vi "AO_master_CorrLoop_PD_2D_v3.vi"() -> ()   [LabVIEW 2018]
uses:
  <userlib>/WaveKit.lib/Controls/Wavefront Corrector states - ONE.ctl
  <userlib>/WaveKit.lib/Classes/WavefrontCorrector/WavefrontCorrector.lvclass
  <userlib>/WaveKit.lib/Classes/WavefrontCorrectorSet/WavefrontCorrectorSet.lvclass
  <vilib>/Analysis/1siggen.llb/Ramp Pattern by Samples.vi
  <vilib>/Utility/file.llb/Read From Spreadsheet File (DBL).vi
  <vilib>/Analysis/1siggen.llb/Ramp Pattern by Delta.vi
  <vilib>/Analysis/NI_AALBase.lvlib
panel:
  in  "Tab Control":T1(tab)
  in  "Flip mirror port":tag="Dev1/ao5"
  in  "interaction matrix file":path=path "D:/SystemAlignment/IM_20200816_1sx2_0p5um.aomi"
  in  "Haso configuration file":path=path "C:/Program Files (x86)/Imagine Optic/Configuration Files/HASO3_first_7364.dat"
  in  "Offset command file":path=path "D:/SystemAlignment/system_aberration_20200627.dat"
  in  "Initial haso file":path=path "D:/SystemAlignment/system_aberration_residual_20200816.has"
  out "# of Phase":i32
  in  "DM configuration file":path=path "C:/Program Files (x86)/Imagine Optic/Configuration Files/WaveFrontCorrector_mirao52-e_0326.dat"
  out "DM Initial State":T2[](array[typedef])
  out "DM ActuatorsNumber":i32
  out "Error out":errorcluster
  in  "EMCCD trigger port":tag="Dev1/port0/line0"
  out "Detector Y Pixels":i32
  out "Detector X Pixels":i32
  out "Return from Initialize":u32
  out "Return from SetTemperature":u32
  out "Calculated Exposure Value":sgl format="%.2f"
  out "Return from CheckTimings":u32
  in  "488 shutter":refnum<k7>(container)
  in  "?":bool
  out "Flip Mirror Status":sgl(ring) items=["EMCCD Camera"=-5, "Wavefront sensor"=1]
  in  "Defocus":bool=TRUE
  in  "Tilts":bool=TRUE
  in  "Max zern num":u32=14
  in  "Density":sgl=0.3 min=0 max=1 format="%#.4f"
  in  "Amplitude":sgl=0.3 min=0 format="%#.4f"
  in  "idxType":enum16{"Wyant", "ANSI"}(ring)=enum."ANSI"
  in  "Zern coeffs file":path=path "D:/SystemAlignment/system_aberration_residual_20200711.txt"
  in  "Diversity Zern Coeffs":enum16{"Manual ", "ZernFile"}(ring)
  out "Zern coeffs (random)":sgl[](array[numeric])
  out "Zern index (random)":i32[](array[numeric])
  in  "Initial Zern Coeffs":enum16{"Manual ", "Random"}(ring)
  in  "Exp Repeat Num":i32=1
  in  "Index 5":i32[](array[numeric])=[3, 4, 5, 6, 7, 8]
  in  "Coeffs 4":sgl[](array[numeric])=[0.5, -0.2, 0.0, 0.0, 0.0, 0.0]
  in  "Index 4":i32[](array[numeric])=[3, 4, 5, 6, 7, 8]
  in  "Coeffs 3":sgl[](array[numeric])=[0.0, -0.2, 0.5, 0.0, 0.0, 0.0]
  in  "Index 3":i32[](array[numeric])=[3, 4, 5, 6, 7, 8]
  in  "Coeffs 2":sgl[](array[numeric])=[0.5, 0.2, 0.0, 0.0, 0.0, 0.0]
  in  "Index 2":i32[](array[numeric])=[3, 4, 5, 6, 7, 8]
  in  "Coeffs 5":sgl[](array[numeric])=[0.0, 0.2, 0.5, 0.0, 0.0, 0.0]
  in  "Zern index initial":i32[](array[numeric])=[3, 5, 6, 7, 12]
  in  "Zern coeffs initial":sgl[](array[numeric])=[0.0, 0.2, 0.0, 0.3, 0.0]
  out "Img Num Used":dbl[](array[numeric])
  out "Corrected IQM":dbl
  out "Recon Img Num":u32=2
  out "Current Exp Num":u32=2
  in  "Auto Stop":bool=TRUE
  in  "Feedback Type":T3(ring)=enum."One Step Feedback"
  in  "Initial Phase Num":u32=2
  out "RMSE Value":dbl
  out "Recon Time (s)":dbl
  in  "File Base Name":string="beads"
  in  "Images/phase":i32=1
  in  "Exposure time (s)":dbl=0.02
  in  "Div Phase Num":i32=5
  in  "Metrics Type":T4(ring)=enum."norm DCT  - spectral domain 3: 0~r0"
  in  "Apply Defocus":bool
  in  "PD Correction":bool=TRUE
  in  "Num for average":u32=1
  in  "Zernike Index Limit":u32=20
  in  "Max Iteration Num":u32=10
  in  "Gamma Value":dbl=1e-10
  in  "Crop Size of image":u32=512
  in  "Background Value":dbl=300.0
  in  "Show Input":bool
  in  "Show Recon":bool=TRUE
  in  "Use GPU":bool=TRUE
  out "Cooling":i32
  in  "Trigger":u32(ring)=1 items=["Internal", "External"]
  in  "Cooler set to Temperature":i32=-60
  in  "Initialize EMCCD?":bool=TRUE
  in  "Turn off EMCCD when finished?":bool
  in  "Main Path":path=path "D:/Data"
  in  "Subfolder":string="Test1"
  in  "Folder Name":string="Test"
  out "Groundtruth IQM":dbl
  out "Aberrated IQM":dbl
  out "All IQM":dbl[](array[numeric])
  in  "Final Phase Num":u32=3
  out "Output path":path=path "D:/Data"
  out "Log File Path":path
  # "AO correction loop based on phase diversity: 2D image case (last update: 20200821)\nVersion 3: A combination of LabVIEW, MATLAB (EMCCD controlled by LabVIEW) for sensorless AO with IQM feedback , modified from Version 2. New updates:\n1) re-organize user interface, reform program design (functions modularized)\n2) set flipping mirror to EMCCD once program runs. \n3) add choice for intial diversity phase # and/or option for not doing IQM feed back.\n4) make batch experiment work, record settings as log file"
  # "How to use\n1) Set Flip mirror to EMCCD (AO_mini_stage and shutter control.vi);\n2) Run this VI;\n3) When cooling gets to -55, the system start to acquire data."
  # "Bugs: \n1) when run this vi first time, there is big shift between diversity images. If repeat, then shift disappears.\n2) diversity image number is not controllable, always output 5 images."
  # "Andor Status"
  # "Manual input"
  # "Random input"
  # "Manual input sequence"
  # "File input"
  # "Path and File Name"
  # "Andor EMCCD Settings"
  # "AO Correction Settings"
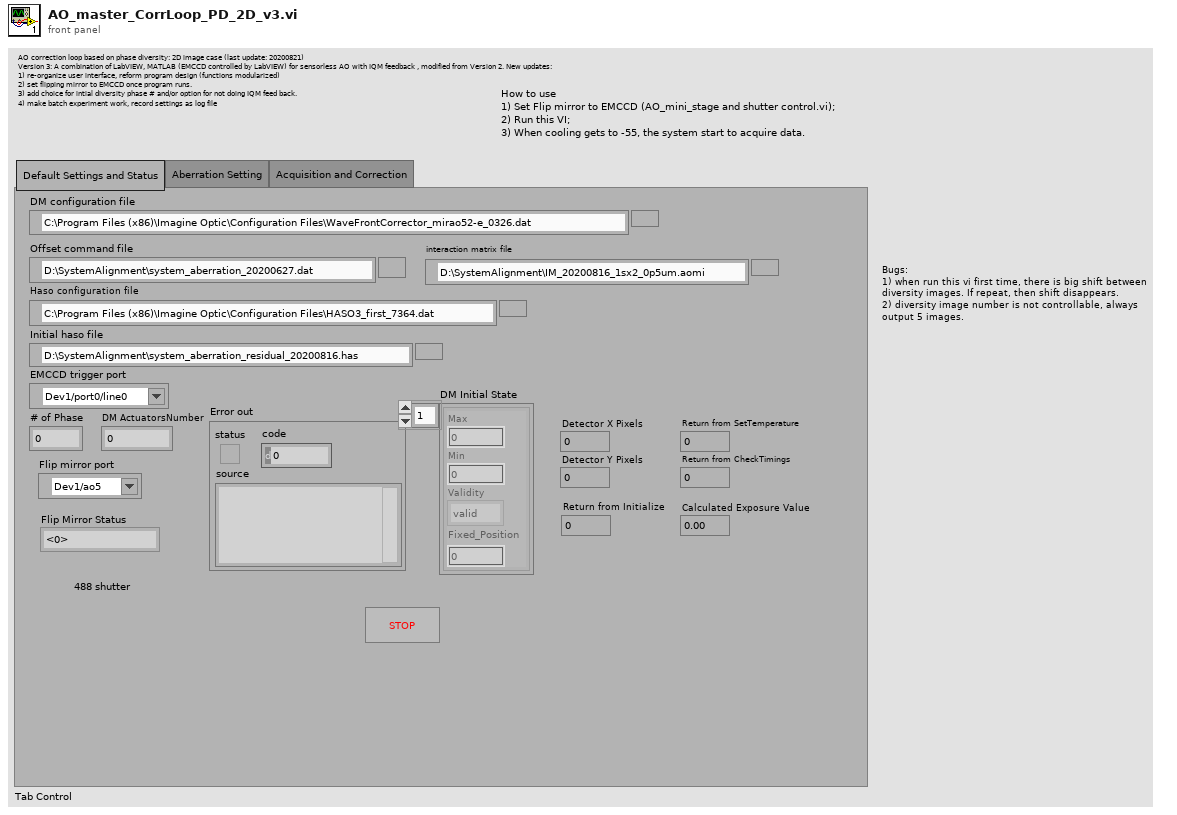
[diagram p1: front panel]
types:
  T1 = enum32{"Default Settings and Status", "Aberration Setting", "Acquisition and Correction"}
  T2 = typedef "Wavefront Corrector states - ONE.ctl" = cluster{"Max":sgl, "Min":sgl, "Validity":enum16{"valid", "fixed", "invalid"}, "Fixed_Position":sgl}
  T3 = enum16{"Single Correction", "One Step Feedback", "Progressive Feedback"}
  T4 = enum16{" ", "max intensity", "mean intensity", "RMS contrast", "sharpness - image domain", "sharpness - spectral domain 1: 0~r0", "sharpness - spectral domain 2: 0.1*r0~0.5*r0", "norm DCT  - spectral domain 3: 0~r0"}
  T5 = typedef "Error Code Enum typedef.ctl" = enum32{"N/A (0)", "DRV_ERROR_CODES", "DRV_SUCCESS", "DRV_VXDNOTINSTALLED", "DRV_ERROR_SCAN", "DRV_ERROR_CHECK_SUM", "DRV_ERROR_FILELOAD", "DRV_UNKNOWN_FUNC", "DRV_ERROR_VXD_INIT", "DRV_ERROR_ADDRESS", "DRV_ERROR_PAGELOCK", "DRV_ERROR_PAGEUNLOCK", "DRV_ERROR_BOARDTEST", "DRV_ERROR_ACK", "DRV_ERROR_UP_FIFO", "DRV_ERROR_PATTERN", "N/A (16)", "DRV_ACQUISITION_ERRORS", "DRV_ACQ_BUFFER", "DRV_ACQ_DOWNFIFO_FULL", "DRV_PROC_UNKONWN_INSTRUCTION", "DRV_ILLEGAL_OP_CODE", "DRV_KINETIC_TIME_NOT_MET", "DRV_ACCUM_TIME_NOT_MET", "DRV_NO_NEW_DATA", "N/A (25)", "DRV_SPOOLERROR", "N/A (27)", "N/A (28)", "N/A (29)", "N/A (30)", "N/A (31)", "N/A (32)", "DRV_TEMPERATURE_CODES", "DRV_TEMPERATURE_OFF", "DRV_TEMPERATURE_NOT_STABILIZED", "DRV_TEMPERATURE_STABILIZED", "DRV_TEMPERATURE_NOT_REACHED", "DRV_TEMPERATURE_OUT_RANGE", "DRV_TEMPERATURE_NOT_SUPPORTED", "DRV_TEMPERATURE_DRIFT", "N/A (41)", "N/A (42)", "N/A (43)", "N/A (44)", "N/A (45)", "N/A (46)", "N/A (47)", "N/A (48)", "DRV_GENERAL_ERRORS", "DRV_INVALID_AUX", "DRV_COF_NOTLOADED", "DRV_FPGAPROG", "DRV_FLEXERROR", "DRV_GPIBERROR", "N/A (55)", "N/A (56)", "N/A (57)", "N/A (58)", "N/A (59)", "N/A (60)", "N/A (61)", "N/A (62)", "N/A (63)", "DRV_DATATYPE", "DRV_DRIVER_ERRORS", "DRV_P1INVALID", "DRV_P2INVALID", "DRV_P3INVALID", "DRV_P4INVALID", "DRV_INIERROR", "DRV_COFERROR", "DRV_ACQUIRING", "DRV_IDLE", "DRV_TEMPCYCLE", "DRV_NOT_INITIALIZED", "DRV_P5INVALID", "DRV_P6INVALID", "DRV_INVALID_MODE", "DRV_INVALID_FILTER", "DRV_I2CERRORS", "DRV_I2CDEVNOTFOUND", "DRV_I2CTIMEOUT", "DRV_P7INVALID", "N/A (84)", "N/A (85)", "N/A (86)", "N/A (87)", "N/A (88)", "N/A (89)", "DRV_IOCERROR", "DRV_VRMVERSIONERROR"}
  T6 = typedef "NI_Matrix.lvlib/RealMatrix.ctl" = dbl[][]
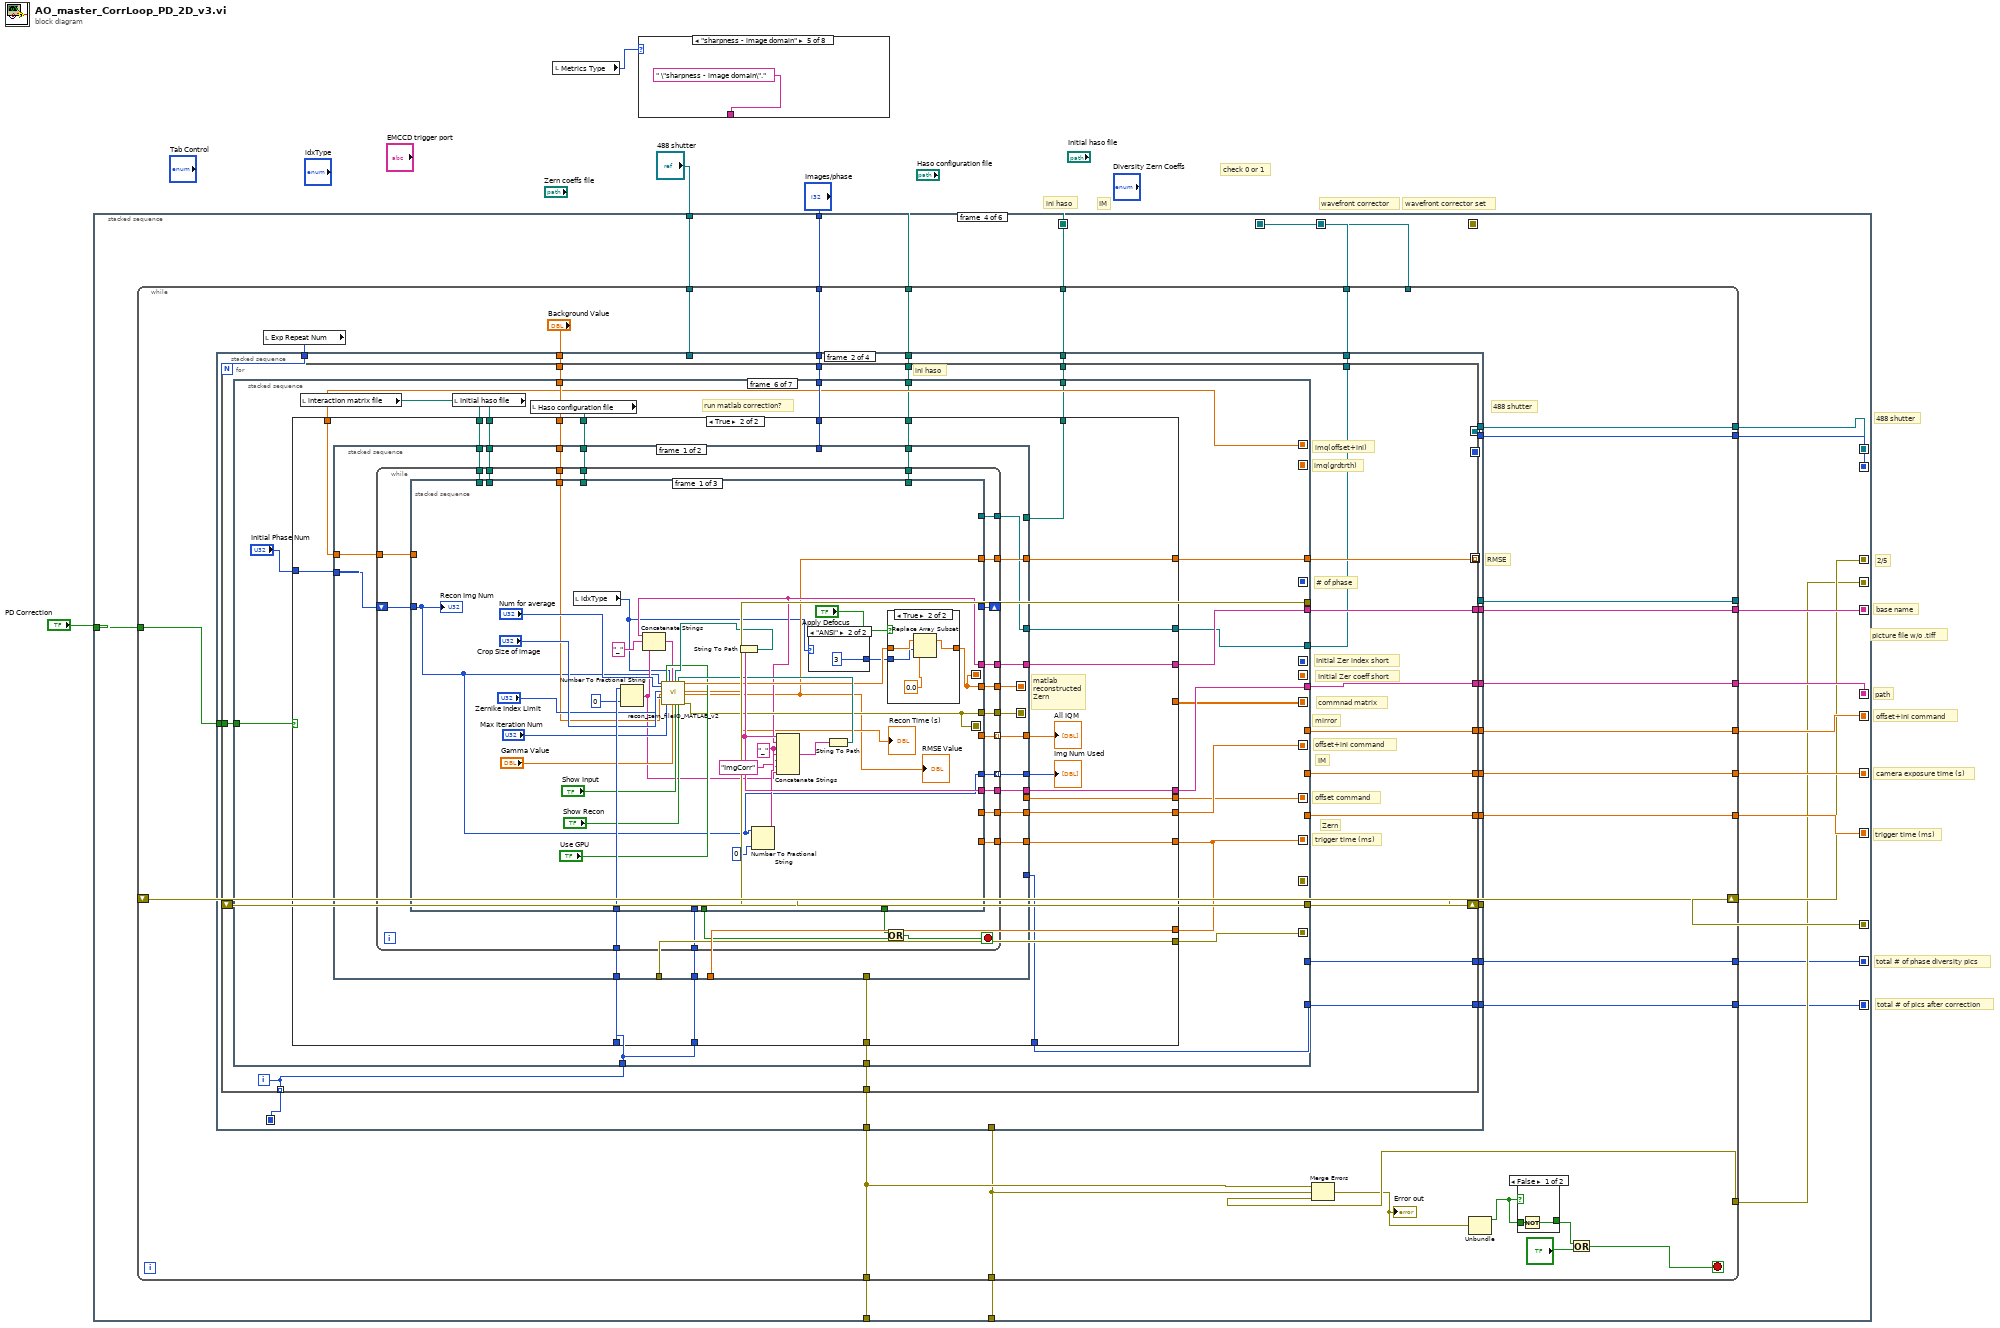
[diagram p0: block diagram]
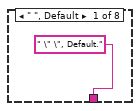
[diagram p2: hidden frame]
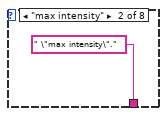
[diagram p3: hidden frame]
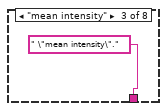
[diagram p4: hidden frame]
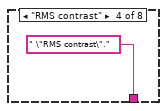
[diagram p5: hidden frame]
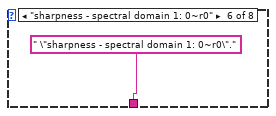
[diagram p6: hidden frame]
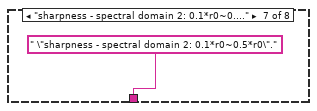
[diagram p7: hidden frame]
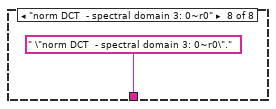
[diagram p8: hidden frame]
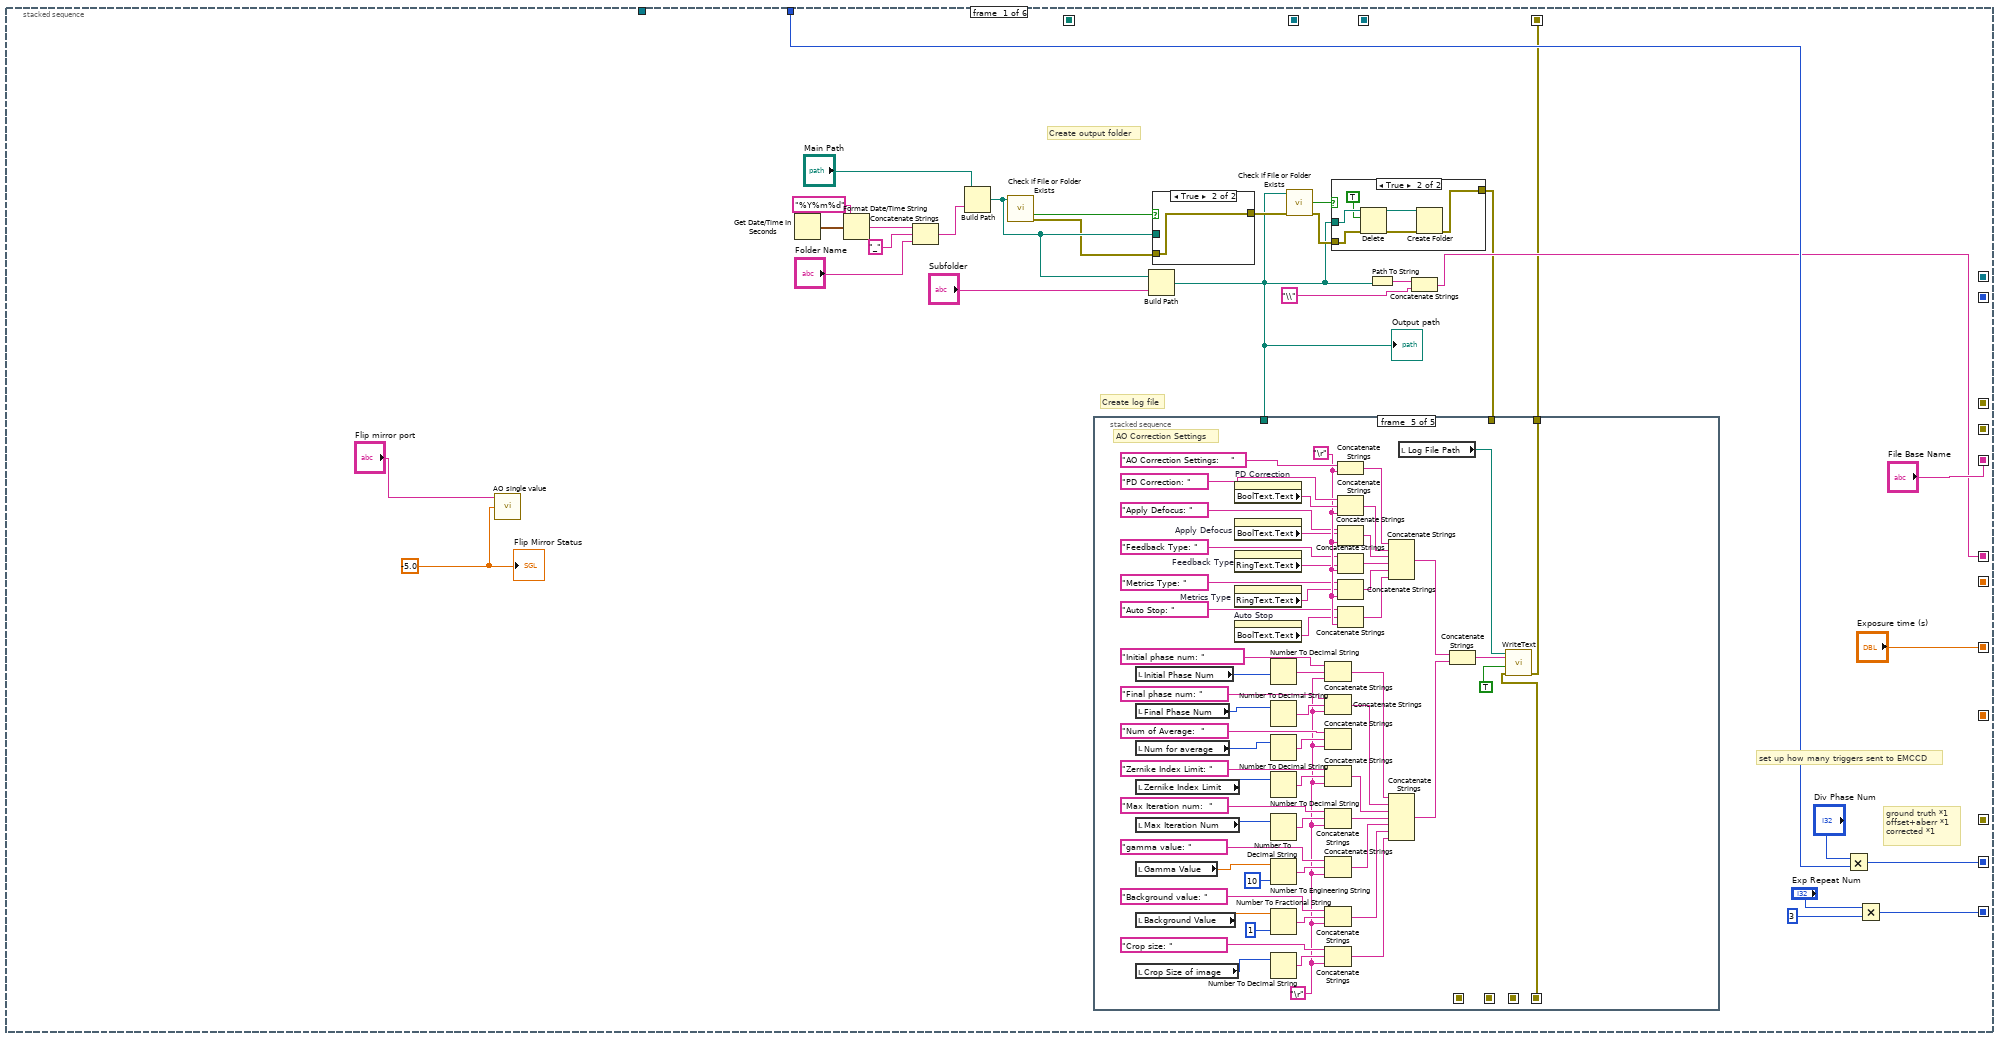
[diagram p9: hidden frame]
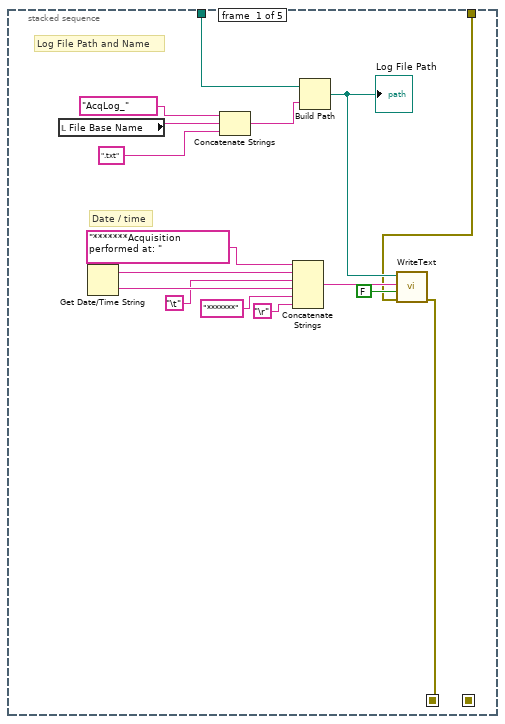
[diagram p10: hidden frame]
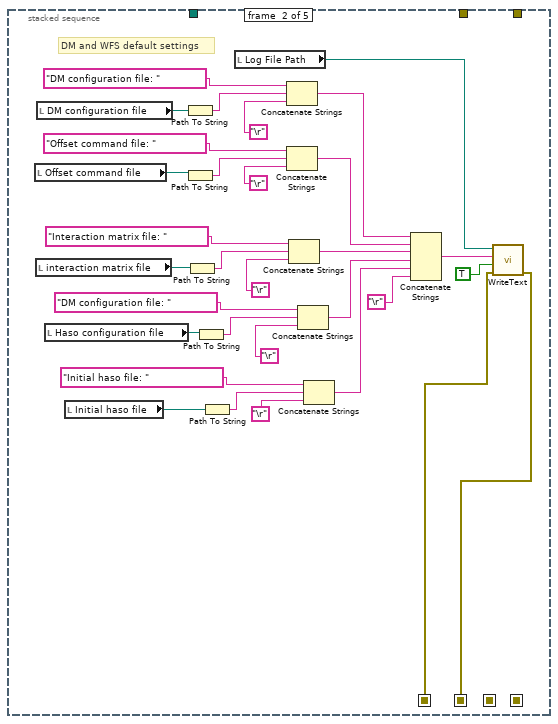
[diagram p11: hidden frame]
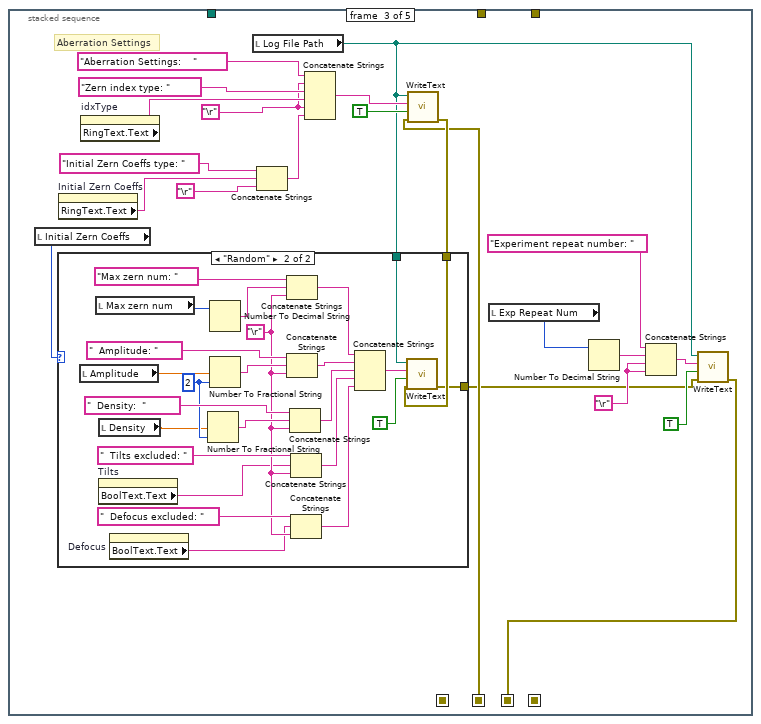
[diagram p12: hidden frame]
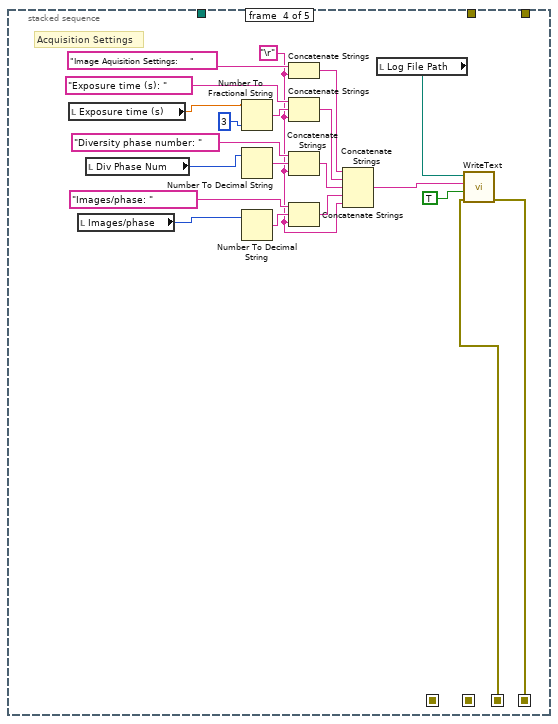
[diagram p14: hidden frame]
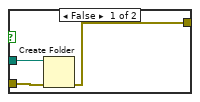
[diagram p15: hidden frame]
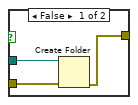
[diagram p16: hidden frame]
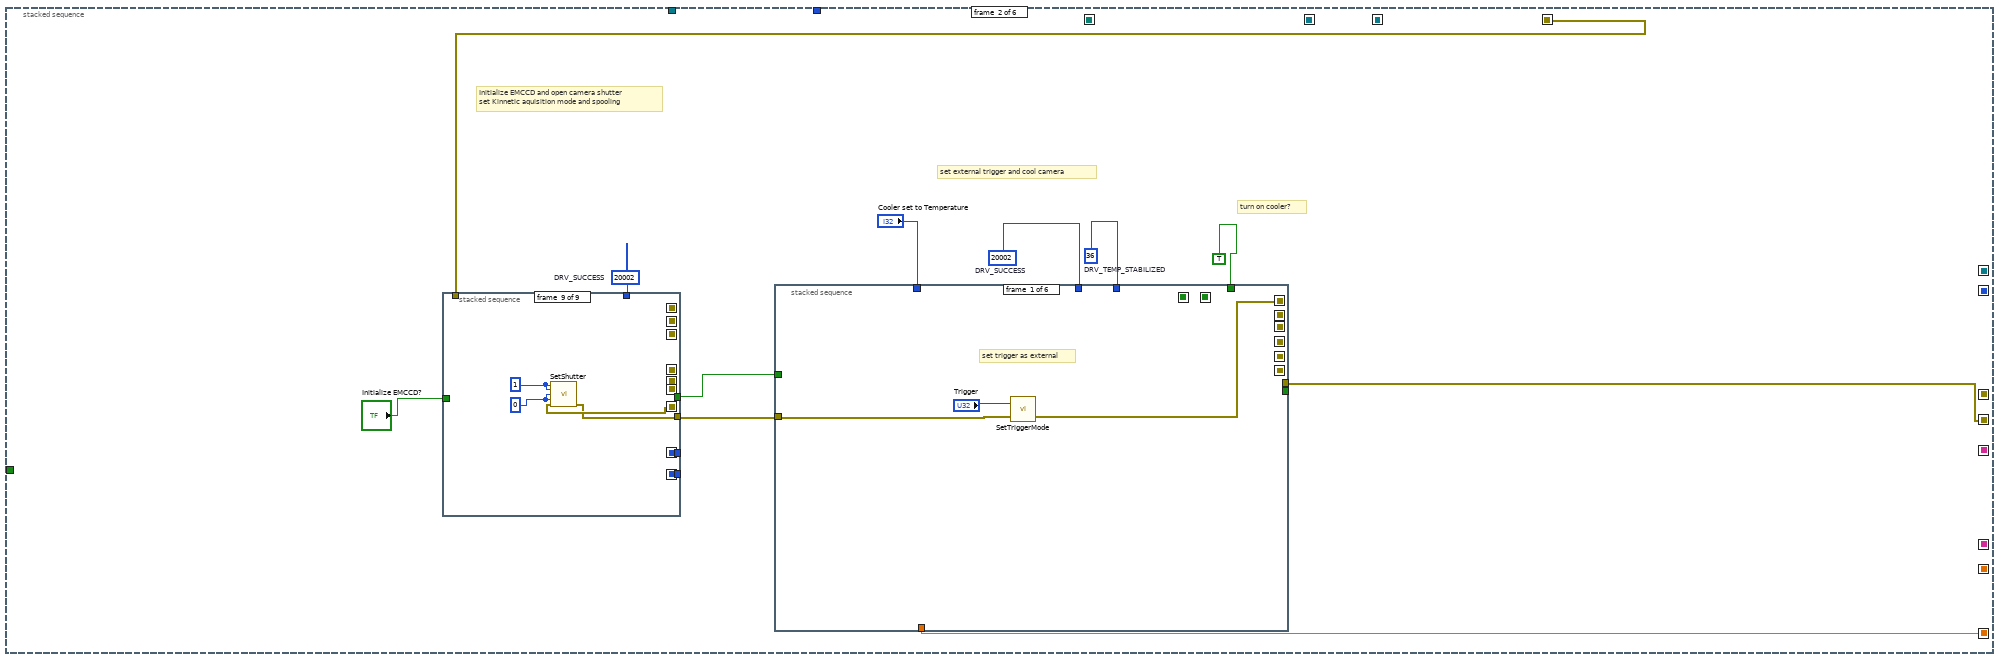
[diagram p17: hidden frame]
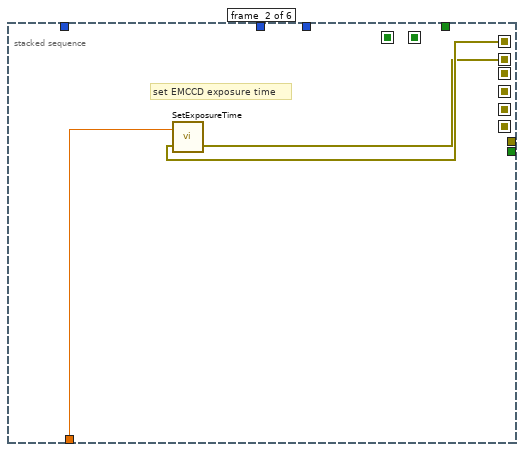
[diagram p18: hidden frame]
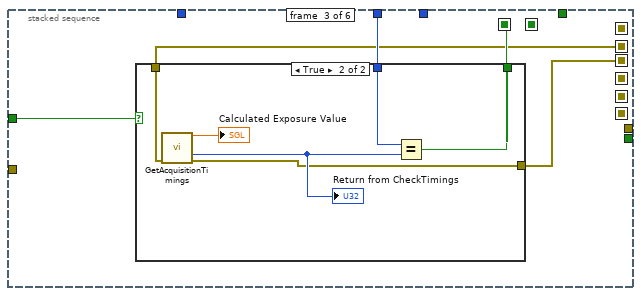
[diagram p19: hidden frame]
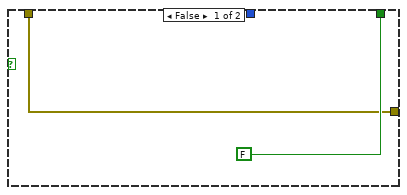
[diagram p20: hidden frame]
diagram:
  # "2/5"
  # "total # of phase diversity pics"
  # "picture file w/o .tiff"
  # "total # of pics after correction"
  # "wavefront corrector set"
  # "wavefront corrector"
  # "488 shutter"
  # "trigger time (ms)"
  # "offset+ini command"
  # "camera exposure time (s)"
  # "IM"
  # "ini haso"
  # "path"
  # "base name"
  # "check 0 or 1"
  n1 = stacked-sequence {
    seq-local: [w14 _ _ _ _ _] -> [_ _ _ w364 _ _]
    seq-local: ["File Base Name" _ _ _ _ _] -> [_ _ _ w363 _ _]
    seq-local: [_ _ w345 _ _ _] -> [_ _ _ w346 _ _]
    seq-local: ["Exposure time (s)" _ _ _ _ _] -> [_ w226 _ w362 _ _]
    seq-local: [_ _ w331 _ _ _] -> [_ _ _ w351 _ _]
    seq-local: [_ _ _ w361 _ _] -> [_ _ _ _ _ _]
    seq-local: [_ _ _ w360 _ _] -> [_ _ _ _ _ _]
    seq-local: [_ _ _ w359 _ _] -> [_ _ _ _ _ w911]
    seq-local: [_ _ _ w354 _ _] -> [_ _ _ _ _ _]
    seq-local: [_ _ _ w357 _ _] -> [_ _ _ _ _ _]
    seq-local: [_ _ w330 _ _ _] -> [_ _ _ w352 _ w913]
    seq-local: [_ _ w329 _ _ _] -> [_ _ _ w350 _ w912]
    seq-local: [w31 _ _ _ _ _] -> [_ _ _ w347 _ _]
    seq-local: [_ w227 _ _ _ _] -> [_ _ w328 w349 _ _]
    seq-local: [w30 _ _ _ _ _] -> [_ _ _ w348 _ _]
    seq-local: [w6 _ _ _ _ _] -> [_ w223 _ _ _ _]
    tunnel: "Images/phase" -> [w29 _ _ w365 _ _]
    tunnel: "PD Correction" -> [_ _ _ w358 _ _]
    tunnel: [_ _ _ w356 _ _] -> _
    tunnel: [_ _ _ w355 _ _] -> _
    tunnel: "488 shutter" -> [_ _ _ w353 _ w914]
    frame #0 {
      w12 = -5.0
      # "Create log file"
      # "Create output folder"
      # "set up how many triggers sent to EMCCD"
      # "ground truth *1\noffset+aberr *1\ncorrected *1"
      n2 = call "AO single value.vi"("data"=w12, "physical channels"="Flip mirror port") -> ()  [unwired: 1 in, 1 out]
      n3 = Get Date/Time In Seconds() -> (seconds since 1Jan1904=w24:timestamp)
      n4 = Format Date/Time String(time format string (%c)="%Y%m%d", seconds (now)=w24) -> (date/time string=w25:string)  [unwired: 1 in]
      n5 = Concatenate Strings(w25, "_", "Folder Name") -> (w26:string)
      n6 = Build Path(base path="Main Path", name or relative path=w26) -> (appended path=w28:path)
      n7 = call <vilib>:"Check if File or Folder Exists.vi"("path"=w28) -> ("error out"=w11:errorcluster, "file or folder exists?"=w22:bool)  [unwired: 8 in, 1 out]
      n8 = Build Path(base path=w28, name or relative path="Subfolder") -> (appended path=w5:path)
      "Output path" <- w5
      n9 = case shown="True" w22 {
        tunnel: w28 -> [w221 _]
        tunnel: w11 -> [w220 w222]
        tunnel: [w219 w222] -> w10
        frame False {
          n10 = Create Folder(path (use dialog)=w221, error in=w220) -> (error out=w219:errorcluster)  [unwired: 1 in, 2 out]
        }
        frame True {
        }
      }
      n11 = call <vilib>:"Check if File or Folder Exists.vi"("error in (no error)"=w10, "path"=w5) -> ("error out"=w27:errorcluster, "file or folder exists?"=w23:bool)  [unwired: 7 in, 1 out]
      n12 = case shown="True" w23 {
        tunnel: w5 -> [w212 w217]
        tunnel: w27 -> [w211 w218]
        tunnel: [w210 w213] -> w7
        frame False {
          n13 = Create Folder(path (use dialog)=w212, error in=w211) -> (error out=w210:errorcluster)  [unwired: 1 in, 2 out]
        }
        frame True {
          n14 = Delete(path (use dialog)=w217, entire hierarchy (F)=TRUE, error in=w218) -> (deleted path=w215:path, error out=w214:errorcluster)  [unwired: 2 in, 1 out]
          n15 = Create Folder(path (use dialog)=w215, error in=w214) -> (error out=w213:errorcluster)  [unwired: 1 in, 2 out]
        }
      }
      n16 = stacked-sequence {
        seq-local: [w36 _ _ _ _] -> [_ w52 _ _ _]
        seq-local: [_ w51 _ _ _] -> [_ _ w98 _ _]
        seq-local: [_ _ w85 _ _] -> [_ _ _ w133 _]
        seq-local: [_ _ _ w132 _] -> [_ _ _ _ w151]
        tunnel: w7 -> [w37 _ _ _ _]
        tunnel: [_ _ _ _ w195] -> w6
        tunnel: w5 -> [w35 _ _ _ _]
        frame #0 {
          # "Date / time"
          # "Log File Path and Name"
          n17 = local read "File Base Name"() -> (w48:string)
          n18 = Get Date/Time String() -> (date string=w45:string, time string=w44:string)  [unwired: 3 in]
          n19 = Concatenate Strings("AcqLog_", w48, ".txt") -> (w50:string)
          n20 = Concatenate Strings("*******Acquisition performed at: ", w45, "\t", w44, "*******", "\r") -> (w40:string)
          n21 = Build Path(base path=w35, name or relative path=w50) -> (appended path=w38:path)
          "Log File Path" <- w38
          n22 = call "WriteText.vi"("error in (no error)"=w37, "Appending"=FALSE, "Input Text"=w40, "File Path"=w38) -> ("error out"=w36:errorcluster)  [unwired: 7 in]
        }
        frame #1 {
          # "DM and WFS default settings"
          n23 = local read "Offset command file"() -> (w74:path)
          n24 = local read "interaction matrix file"() -> (w63:path)
          n25 = local read "DM configuration file"() -> (w79:path)
          n26 = local read "Haso configuration file"() -> (w62:path)
          n27 = local read "Initial haso file"() -> (w61:path)
          n28 = Path To String(path=w79) -> (string=w78:string)
          n29 = Path To String(path=w74) -> (string=w75:string)
          n30 = Path To String(path=w63) -> (string=w70:string)
          n31 = Path To String(path=w62) -> (string=w67:string)
          n32 = Path To String(path=w61) -> (string=w64:string)
          n33 = local read "Log File Path"() -> (w60:path)
          n34 = Concatenate Strings("DM configuration file: ", w78, "\r") -> (w58:string)
          n35 = Concatenate Strings("Offset command file: ", w75, "\r") -> (w57:string)
          n36 = Concatenate Strings("Interaction matrix file: ", w70, "\r") -> (w59:string)
          n37 = Concatenate Strings("DM configuration file: ", w67, "\r") -> (w55:string)
          n38 = Concatenate Strings("Initial haso file: ", w64, "\r") -> (w56:string)
          n39 = Concatenate Strings(w58, w57, w59, w55, w56, "\r") -> (w53:string)
          n40 = call "WriteText.vi"("error in (no error)"=w52, "Appending"=TRUE, "Input Text"=w53, "File Path"=w60) -> ("error out"=w51:errorcluster)  [unwired: 7 in]
        }
        frame #2 {
          w87 = "\r"
          w82 = "\r"
          # "Aberration Settings"
          n41 = local read "Initial Zern Coeffs"() -> (w93:enum16{"Manual ", "Random"})
          n42 = property on="Initial Zern Coeffs" class="Enum (strict)"() -> ("RingText.Text"=w95:string)  [unwired: 2 in, 2 out]
          n43 = property on="idxType" class="Enum (strict)"() -> ("RingText.Text"=w99:string)  [unwired: 2 in, 2 out]
          n44 = local read "Log File Path"() -> (w84:path)
          n45 = Concatenate Strings("Initial Zern Coeffs type: ", w95, "\r") -> (w94:string)
          n46 = Concatenate Strings("Aberration Settings:    ", w82, "Zern index type: ", w99, w82, w94) -> (w101:string)
          n47 = call "WriteText.vi"("error in (no error)"=w98, "Appending"=TRUE, "Input Text"=w101, "File Path"=w84) -> ("error out"=w100:errorcluster)  [unwired: 7 in]
          n48 = case shown="\"Random\"" w93 {
            tunnel: w84 -> [_ w125]
            tunnel: w100 -> [w104 w124]
            tunnel: [w104 w123] -> w86
            frame "Manual ", Default {
            }
            frame "Random" {
              w116 = 2
              w109 = "\r"
              n49 = local read "Amplitude"() -> (w127:sgl)
              n50 = local read "Max zern num"() -> (w126:u32)
              n51 = local read "Density"() -> (w115:sgl)
              n52 = property on="Tilts" class="Bool (strict)"() -> ("BoolText.Text"=w108:string)  [unwired: 2 in, 2 out]
              n53 = property on="Defocus" class="Bool (strict)"() -> ("BoolText.Text"=w107:string)  [unwired: 2 in, 2 out]
              n54 = Number To Fractional String(number=w115, precision (6)=w116) -> (F-format string=w117:string)  [unwired: 2 in]
              n55 = Number To Decimal String(number=w126) -> (decimal integer string=w121:string)  [unwired: 1 in]
              n56 = Number To Fractional String(number=w127, precision (6)=w116) -> (F-format string=w119:string)  [unwired: 2 in]
              n57 = Concatenate Strings("Max zern num: ", w121, w109) -> (w114:string)
              n58 = Concatenate Strings("  Amplitude: ", w119, w109) -> (w113:string)
              n59 = Concatenate Strings("  Density:  ", w117, w109) -> (w112:string)
              n60 = Concatenate Strings("  Tilts excluded: ", w108, w109) -> (w105:string)
              n61 = Concatenate Strings("  Defocus excluded: ", w107, w109) -> (w106:string)
              n62 = Concatenate Strings(w114, w113, w112, w105, w106) -> (w128:string)
              n63 = call "WriteText.vi"("error in (no error)"=w124, "Appending"=TRUE, "Input Text"=w128, "File Path"=w125) -> ("error out"=w123:errorcluster)  [unwired: 7 in]
            }
          }
          n64 = local read "Exp Repeat Num"() -> (w89:i32)
          n65 = Number To Decimal String(number=w89) -> (decimal integer string=w90:string)  [unwired: 1 in]
          n66 = Concatenate Strings("Experiment repeat number: ", w90, w87, w87) -> (w91:string)
          n67 = call "WriteText.vi"("error in (no error)"=w86, "Appending"=TRUE, "Input Text"=w91, "File Path"=w84) -> ("error out"=w85:errorcluster)  [unwired: 7 in]
        }
        frame #3 {
          w130 = "\r"
          # "Acquisition Settings"
          n68 = local read "Exposure time (s)"() -> (w135:dbl)
          n69 = local read "Images/phase"() -> (w137:i32)
          n70 = local read "Div Phase Num"() -> (w139:i32)
          n71 = Number To Fractional String(number=w135, precision (6)=3) -> (F-format string=w131:string)  [unwired: 2 in]
          n72 = Number To Decimal String(number=w139) -> (decimal integer string=w148:string)  [unwired: 1 in]
          n73 = Number To Decimal String(number=w137) -> (decimal integer string=w147:string)  [unwired: 1 in]
          n74 = Concatenate Strings("Image Aquisition Settings:    ", w130) -> (w146:string)
          n75 = Concatenate Strings("Exposure time (s): ", w131, w130) -> (w145:string)
          n76 = Concatenate Strings("Diversity phase number: ", w148, w130) -> (w144:string)
          n77 = Concatenate Strings("Images/phase: ", w147, w130) -> (w143:string)
          n78 = Concatenate Strings(w146, w145, w144, w143, w130) -> (w136:string)
          n79 = local read "Log File Path"() -> (w149:path)
          n80 = call "WriteText.vi"("error in (no error)"=w133, "Appending"=TRUE, "Input Text"=w136, "File Path"=w149) -> ("error out"=w132:errorcluster)  [unwired: 7 in]
        }
        frame #4 {
          w162 = "\r"
          w192 = "\r"
          # "AO Correction Settings"
          n81 = local read "Initial Phase Num"() -> (w201:u32)
          n82 = local read "Final Phase Num"() -> (w199:u32)
          n83 = local read "Num for average"() -> (w176:u32)
          n84 = local read "Zernike Index Limit"() -> (w173:u32)
          n85 = local read "Max Iteration Num"() -> (w170:u32)
          n86 = local read "Gamma Value"() -> (w198:dbl)
          n87 = local read "Background Value"() -> (w166:dbl)
          n88 = local read "Crop Size of image"() -> (w163:u32)
          n89 = property on="PD Correction" class="Bool (strict)"() -> ("BoolText.Text"=w194:string)  [unwired: 2 in, 2 out]
          n90 = property on="Apply Defocus" class="Bool (strict)"() -> ("BoolText.Text"=w191:string)  [unwired: 2 in, 2 out]
          n91 = property on="Feedback Type" class="Enum (strict)"() -> ("RingText.Text"=w189:string)  [unwired: 2 in, 2 out]
          n92 = property on="Metrics Type" class="Enum (strict)"() -> ("RingText.Text"=w187:string)  [unwired: 2 in, 2 out]
          n93 = property on="Auto Stop" class="Bool (strict)"() -> ("BoolText.Text"=w185:string)  [unwired: 2 in, 2 out]
          n94 = Number To Decimal String(number=w201) -> (decimal integer string=w207:string)  [unwired: 1 in]
          n95 = Number To Decimal String(number=w199) -> (decimal integer string=w206:string)  [unwired: 1 in]
          n96 = Number To Decimal String(number=w176) -> (decimal integer string=w178:string)  [unwired: 1 in]
          n97 = Number To Decimal String(number=w173) -> (decimal integer string=w175:string)  [unwired: 1 in]
          n98 = Number To Decimal String(number=w170) -> (decimal integer string=w172:string)  [unwired: 1 in]
          n99 = Number To Engineering String(2:10, 4:w198) -> (0:w196:string)  [unwired: 2 in]
          n100 = Number To Fractional String(number=w166, precision (6)=1) -> (F-format string=w167:string)  [unwired: 2 in]
          n101 = Number To Decimal String(number=w163) -> (decimal integer string=w165:string)  [unwired: 1 in]
          n102 = Concatenate Strings("Initial phase num: ", w207, w162) -> (w161:string)
          n103 = Concatenate Strings("Final phase num: ", w206, w162) -> (w160:string)
          n104 = Concatenate Strings("Num of Average:  ", w178, w162) -> ()  [unwired: 1 out]
          n105 = Concatenate Strings("Zernike Index Limit: ", w175, w162) -> (w159:string)
          n106 = Concatenate Strings("Max Iteration num:  ", w172, w162) -> (w155:string)
          n107 = Concatenate Strings("gamma value: ", w196, w162) -> (w156:string)
          n108 = Concatenate Strings("Background value: ", w167, w162) -> (w157:string)
          n109 = Concatenate Strings("Crop size: ", w165, w162) -> (w158:string)
          n110 = Concatenate Strings("AO Correction Settings:    ", w192) -> (w205:string)
          n111 = Concatenate Strings("PD Correction: ", w194, w192) -> (w183:string)
          n112 = Concatenate Strings("Apply Defocus: ", w191, w192) -> (w182:string)
          n113 = Concatenate Strings("Feedback Type: ", w189, w192) -> (w179:string)
          n114 = Concatenate Strings("Metrics Type: ", w187, w192) -> (w180:string)
          n115 = Concatenate Strings("Auto Stop: ", w185, w192) -> (w181:string)
          n116 = Concatenate Strings(w205, w183, w182, w179, w180, w181) -> (w153:string)
          n117 = Concatenate Strings(w161, w160, w159, w155, w156, w157, w158) -> (w152:string)
          n118 = local read "Log File Path"() -> (w208:path)
          n119 = Concatenate Strings(w153, w152) -> (w154:string)
          n120 = call "WriteText.vi"("error in (no error)"=w151, "Appending"=TRUE, "Input Text"=w154, "File Path"=w208) -> ("error out"=w195:errorcluster)  [unwired: 7 in]
        }
      }
      n121 = Path To String(path=w5) -> (string=w16:string)
      n122 = Concatenate Strings(w16, "\\") -> (w14:string)
      n123 = Multiply(x="Div Phase Num", y=w29) -> (x*y=w30:i32)
      n124 = Multiply(x="Exp Repeat Num", y=3) -> (x*y=w31:i32)
      "Flip Mirror Status" <- w12
    }
    frame #1 {
      w229 = 36  # DRV_TEMP_STABILIZED
      w231 = 20002  # DRV_SUCCESS
      w233 = 20002  # DRV_SUCCESS
      # "turn on cooler?"
      # "set external trigger and cool camera"
      # "Initialize EMCCD and open camera shutter\nset Kinnetic aquisition mode and spooling"
      n125 = stacked-sequence {
        seq-local: [_ _ _ _ _ _ _ w317 _] -> [_ _ _ _ _ _ _ _ _]
        seq-local: [_ _ _ _ _ _ _ w319 _] -> [_ _ _ _ _ _ _ _ _]
        seq-local: [w287 _ _ _ _ _ _ _ _] -> [_ _ w300 _ _ _ _ _ _]
        seq-local: [_ _ w299 _ _ _ _ _ _] -> [_ _ _ w303 _ _ _ _ _]
        seq-local: [_ _ _ w302 _ _ _ _ _] -> [_ _ _ _ w305 _ _ _ _]
        seq-local: [_ _ _ _ w306 _ _ _ _] -> [_ _ _ _ _ w309 _ _ _]
        seq-local: [_ _ _ _ _ w308 _ _ _] -> [_ _ _ _ _ _ w313 _ _]
        seq-local: [_ _ _ _ _ _ w311 _ _] -> [_ _ _ _ _ _ _ w322 _]
        seq-local: [_ _ _ _ _ _ _ w320 _] -> [_ _ _ _ _ _ _ _ w325]
        tunnel: w233 -> [w289 _ _ _ _ _ _ _ _]
        tunnel: [w288 _ _ _ _ _ _ _ _] -> w232
        tunnel: [_ _ _ _ _ _ _ w317 _] -> _
        tunnel: [_ _ _ _ _ _ _ w319 _] -> _
        tunnel: [_ _ _ _ _ _ _ _ w324] -> w228
        tunnel: "Initialize EMCCD?" -> [w286 _ _ _ _ _ _ _ _]
        tunnel: w223 -> [w285 _ _ _ _ _ _ _ _]
        frame #0 {
          # "Initialize EMCCD"
          n126 = case shown="True" w286 {
            tunnel: w289 -> [_ w295]
            tunnel: [TRUE w294] -> w288
            tunnel: [errorcluster {"status"=FALSE, "code"=0, "source"=""} ("Error in 2") w293] -> w287
            tunnel: w285 -> [_ w292]
            frame False {
            }
            frame True {
              n127 = call <userlib>:"Initialize.vi"("error in (no error)"=w292, "directory (\"\")"="" ("directory (\"\")")) -> ("error out"=w293:errorcluster, "DLL error code"=w297:u32)
              "Return from Initialize" <- w297
              n128 = Equal?(x=w295, y=w297) -> (x = y?=w294:bool)
            }
          }
        }
        frame #1 {
          # "It's 2 seconds in andor example vi"
          n129 = Wait (ms)(milliseconds to wait=u32 500) -> ()  [unwired: 1 out]
        }
        frame #2 {
          w301 = u16 4  # ReadMode: Image
          n130 = call <userlib>:"SetReadMode.vi"("error in (no error)"=w300, "mode"=w301) -> ("error out"=w299:errorcluster)  [unwired: 1 out]
        }
        frame #3 {
          w304 = u16 3  # AcquisitionMode: Kinetics
          n131 = call <userlib>:"SetAcquisitionMode.vi"("error in (no error)"=w303, "mode"=w304) -> ("error out"=w302:errorcluster)  [unwired: 1 out]
        }
        frame #4 {
          n132 = call <userlib>:"SetADChannel.vi"("error in (no error)"=w305, "channel"=0) -> ("error out"=w306:errorcluster)  [unwired: 1 out]
        }
        frame #5 {
          w310 = 0
          n133 = call <userlib>:"SetHSSpeed.vi"("error in (no error)"=w309, "index"=w310, "type"=w310) -> ("error out"=w308:errorcluster)  [unwired: 1 in, 1 out]
        }
        frame #6 {
          n134 = call <userlib>:"GetNumberVSSpeeds.vi"("error in (no error)"=w313) -> ("error out"=w312:errorcluster, "number"=w316:i32)  [unwired: 2 in, 1 out]
          n135 = Subtract(x=w316, y=1) -> (x-y=w314:i32)
          n136 = call <userlib>:"SetVSSpeed.vi"("error in (no error)"=w312, "index"=w314) -> ("error out"=w311:errorcluster)  [unwired: 1 out]
        }
        frame #7 {
          w323 = 1
          n137 = call <userlib>:"GetDetector.vi"("error in (no error)"=w322) -> ("error out"=w321:errorcluster, "ypixels"=w318:i32, "xpixels"=w319:i32)  [unwired: 3 in, 1 out]
          "Detector Y Pixels" <- w318
          "Detector X Pixels" <- w319
          n138 = Max & Min(x=w319, y=w318) -> (min(x,y)=w317:i32)  [unwired: 1 out]
          n139 = call <userlib>:"SetImage.vi"("hbin"=w323, "vbin"=w323, "hstart"=w323, "hend"=w317, "vstart"=w323, "vend"=w317, "error in (no error)"=w321) -> ("error out"=w320:errorcluster)  [unwired: 19 in, 1 out]
        }
        frame #8 {
          w326 = 0
          w327 = 1
          n140 = call <userlib>:"SetShutter.vi"("type"=w327, "mode"=w327, "closingtime"=w326, "openingtime"=w326, "error in (no error)"=w325) -> ("error out"=w324:errorcluster)  [unwired: 9 in, 1 out]
        }
      }
      n141 = stacked-sequence {
        seq-local: [_ _ w242 _ _ _] -> [_ _ _ _ _ _]
        seq-local: [_ _ _ w255 _ _] -> [_ _ _ _ _ _]
        seq-local: [w234 _ _ _ _ _] -> [_ w239 _ _ _ _]
        seq-local: [_ w238 _ _ _ _] -> [_ _ w241 _ _ _]
        seq-local: [_ _ w240 _ _ _] -> [_ _ _ w254 _ _]
        seq-local: [_ _ _ w253 _ _] -> [_ _ _ _ w261 _]
        seq-local: [_ _ _ _ w260 _] -> [_ _ _ _ _ w267]
        seq-local: [_ _ _ _ _ w265] -> [_ _ _ _ _ _]
        tunnel: w231 -> [_ _ w244 w258 _ _]
        tunnel: "Cooler set to Temperature" -> [_ _ _ w256 _ w268]
        tunnel: w229 -> [_ _ _ _ _ w269]
        tunnel: [_ _ _ w255 _ _] -> _
        tunnel: w232 -> [_ _ w243 _ _ _]
        tunnel: w228 -> [w235 _ _ _ _ _]
        tunnel: [_ _ _ _ _ w265] -> w227
        tunnel: w226 -> [_ w237 _ _ _ _]
        tunnel: TRUE -> [_ _ _ _ w259 w266]
        frame #0 {
          # "set trigger as external"
          n142 = call <userlib>:"SetTriggerMode.vi"("error in (no error)"=w235, "mode"="Trigger") -> ("error out"=w234:errorcluster)  [unwired: 1 out]
        }
        frame #1 {
          # "set EMCCD exposure time"
          n143 = call <userlib>:"SetExposureTime.vi"("error in (no error)"=w239, "time"=w237) -> ("error out"=w238:errorcluster)  [unwired: 1 out]
        }
        frame #2 {
          n144 = case shown="True" w243 {
            tunnel: w244 -> [_ w250]
            tunnel: [FALSE w252] -> w242
            tunnel: w241 -> [w245 w248]
            tunnel: [w245 w247] -> w240
            frame False {
            }
            frame True {
              n145 = call <userlib>:"GetAcquisitionTimings.vi"("error in (no error)"=w248) -> ("exposure"=→"Calculated Exposure Value":sgl, "DLL error code"=w249:u32, "error out"=w247:errorcluster)  [unwired: 10 in, 2 out]
              "Return from CheckTimings" <- w249
              n146 = Equal?(x=w250, y=w249) -> (x = y?=w252:bool)
            }
          }
        }
        frame #3 {
          # "set camera temperature to -60C"
          n147 = call <userlib>:"SetTemperature.vi"("error in (no error)"=w254, "temperature"=w256) -> ("error out"=w253:errorcluster, "DLL error code"=w257:u32)
          "Return from SetTemperature" <- w257
          n148 = Equal?(x=w258, y=w257) -> (x = y?=w255:bool)
        }
        frame #4 {
          # "turn on cooler"
          n149 = case shown="True" w259 {
            tunnel: w261 -> [w262 w264]
            tunnel: [w262 w263] -> w260
            frame False {
            }
            frame True {
              n150 = call <userlib>:"CoolerON.vi"("error in (no error)"=w264) -> ("error out"=w263:errorcluster)  [unwired: 1 in, 1 out]
            }
          }
        }
        frame #5 {
          # "wait the camera to cool down,\nwill not move forward untill the temperature reach 60C"
          n151 = case shown="True" w266 {
            tunnel: w269 -> [_ w274]
            tunnel: w268 -> [_ w273]
            tunnel: w267 -> [w270 w272]
            tunnel: [w270 w271] -> w265
            frame False {
            }
            frame True {
              n152 = while {
                tunnel: w274 -> [w283]
                tunnel: w273 -> [w278]
                tunnel: w272 -> [w281]
                tunnel: [w280] -> w271
                stop <- w275 continue-if-true
                n153 = Wait Until Next ms Multiple(millisecond multiple=u32 500) -> ()  [unwired: 1 out]
                n154 = call <userlib>:"GetTemperature.vi"("error in (no error)"=w281) -> ("error out"=w280:errorcluster, "status"=w282:T5, "temperature"=w276:i32)  [unwired: 3 in, 1 out]
                "Cooling" <- w276
                n155 = Add(x=w278, y=5) -> (x+y=w277:i32)
                n156 = Not Equal?(x=w283, y=w282) -> ()  [unwired: 1 out]
                n157 = Greater?(x=w276, y=w277) -> (0:w275:bool)
              }
            }
          }
        }
      }
    }
    frame #2 {
      # "Initialize CASAO"
      n158 = call <userlib>:"LVClass_WavefrontCorrectorSet ctor.vi"("WavefrontCorrectorSet in"=refnum<class "WavefrontCorrectorSet.lvclass"> refnum, "PathToWavefrontCorrectorSetupFile"="DM configuration file", "error in (no error)"=w328) -> ("WavefrontCorrectorSet out"=w335:refnum<class "WavefrontCorrectorSet.lvclass">, "error out"=w344:errorcluster)  [unwired: 11 in]
      n159 = call <userlib>:"LVClass_WavefrontCorrector ctor.vi"("WavefrontCorrector in"=refnum<class "WavefrontCorrector.lvclass"> refnum, "PathToWavefrontCorrectorSetupFile"="DM configuration file", "error in (no error)"=w344) -> ("WavefrontCorrector out"=w339:refnum<class "WavefrontCorrector.lvclass">, "error out"=w338:errorcluster)  [unwired: 11 in]
      n160 = call <userlib>:"LVClass_WavefrontCorrector Init.vi"("WavefrontCorrector in"=w339, "set_init_state_from_config_file"=TRUE, "error in (no error)"=w338) -> ("WavefrontCorrector out"=w333:refnum<class "WavefrontCorrector.lvclass">, "error out"=w337:errorcluster)  [unwired: 11 in]
      n161 = call <userlib>:"LVClass_WavefrontCorrectorSet get nb of actuators.vi"("WavefrontCorrectorSet in"=w335, "error in (no error)"=w337) -> ("WavefrontCorrectorSet out"=w329:refnum<class "WavefrontCorrectorSet.lvclass">, "ActuatorsNumber"=→"DM ActuatorsNumber":i32, "error out"=w334:errorcluster)  [unwired: 11 in]
      n162 = call <userlib>:"LVClass_WavefrontCorrector Get Current Preferences.vi"("WavefrontCorrector in"=w333, "error in (no error)"=w334) -> ("WavefrontCorrector out"=w330:refnum<class "WavefrontCorrector.lvclass">, "Mirror preferences.Wavefront Corrector State"=→"DM Initial State":T2[], "error out"=w331:errorcluster)  [unwired: 10 in, 1 out]
      n163 = local read "Initial haso file"() -> (w345:path)
    }
    frame #3 {
      n164 = while {
        tunnel: w365 -> [w393]
        tunnel: w364 -> [w392]
        tunnel: w363 -> [w391]
        tunnel: w346 -> [w390]
        tunnel: w362 -> [w389]
        tunnel: [w387] -> w361
        tunnel: [w386] -> w360
        tunnel: w358 -> [w384]
        tunnel: [w383] -> w357
        tunnel: [w382] -> _
        tunnel: [w380] -> w356
        tunnel: [w381] -> w355
        shift-right: [w385] -> w359
        shift-left: w351 -> [w388]
        tunnel: [w379] -> w354
        tunnel: w353 -> [w378]
        tunnel: w352 -> [w377]
        tunnel: w350 -> [_]
        tunnel: w349 -> [w375]
        tunnel: w348 -> [w369]
        tunnel: w347 -> [w368]
        tunnel: w346 -> [w366]
        stop <- w371 stop-if-true
        # "488 shutter"
        # "RMSE"
        n165 = local read "Exp Repeat Num"() -> (w376:i32)
        n166 = stacked-sequence {
          seq-local: [_ w412 _ _] -> [_ _ _ w903]
          seq-local: [_ w411 _ _] -> [_ _ _ _]
          seq-local: [w399 _ _ _] -> [_ _ w899 _]
          seq-local: [w400 _ _ _] -> [_ _ w898 _]
          tunnel: w393 -> [_ w423 _ _]
          tunnel: w392 -> [_ w422 _ w902]
          tunnel: w391 -> [_ w421 _ w901]
          tunnel: w390 -> [_ w420 _ _]
          tunnel: w389 -> [_ w419 _ _]
          tunnel: w388 -> [_ w418 _ _]
          tunnel: [_ w417 _ _] -> w387
          tunnel: [_ w416 _ _] -> w386
          tunnel: [_ w415 _ _] -> w385
          tunnel: w384 -> [_ w414 _ _]
          tunnel: w376 -> [_ w413 _ _]
          tunnel: [_ _ w897 _] -> w382
          tunnel: [_ _ w896 _] -> w383
          tunnel: [_ _ _ w900] -> w380
          tunnel: [_ w410 _ _] -> w381
          tunnel: [w399 _ _ _] -> w379
          tunnel: w378 -> [w398 _ _ _]
          tunnel: w377 -> [_ w409 _ _]
          tunnel: w369 -> [_ w408 _ _]
          tunnel: w368 -> [_ w407 _ _]
          tunnel: "Background Value" -> [_ w406 _ _]
          tunnel: w366 -> [_ w405 _ _]
          frame #0 {
            # "open the shutter of 488nm laser"
            n167 = property class="MG17Motor"(reference=w398, "HWSerialNum"=85819115.0) -> (reference out=w404:refnum<k7>)  [unwired: 1 in, 1 out]
            n168 = invoke class="MG17Motor" method="StartCtrl"(reference=w404) -> (reference out=w402:refnum<k7>)  [unwired: 2 in, 2 out]
            n169 = Wait (ms)(milliseconds to wait=1000) -> ()  [unwired: 1 out]
            n170 = invoke class="MG17Motor" method="SC_Enable"(reference=w402, "lChanID"=0) -> (reference out=w399:refnum<k7>, "lChanID"=w400:i32)  [unwired: 2 in, 2 out]
          }
          frame #1 {
            n171 = for {
              N: w413 -> [_]
              tunnel: w423 -> [w441]
              tunnel: w422 -> [w440]
              tunnel: w421 -> [w439]
              tunnel: w420 -> [w438]
              tunnel: w419 -> [w437]
              tunnel: [w435] -> w417
              tunnel: [w434] -> w416
              tunnel: w414 -> [w432]
              shift-right: [w433] -> w415
              shift-left: w418 -> [w436]
              tunnel: [w431] -> w412 mode=indexing
              tunnel: [w430] -> w411 mode=indexing
              tunnel: [w429] -> w410
              tunnel: w409 -> [w428]
              tunnel: w408 -> [w427]
              tunnel: w407 -> [w426]
              tunnel: w406 -> [w425]
              tunnel: w405 -> [w424]
              i -> [w430]
              # "imq(grdtrth)"
              # "imq(offset+ini)"
              # "# of phase"
              # "trigger time (ms)"
              # "offset+ini command"
              # "Initial Zer coeff short"
              # "Initial Zer index short"
              # "mirror"
              # "Zern"
              # "commnad matrix"
              # "ini haso"
              # "IM"
              # "offset command"
              n172 = stacked-sequence {
                seq-local: [_ w457 _ _ _ _ _] -> [_ _ w475 _ w611 w669 _]
                seq-local: [_ _ w473 _ _ _ _] -> [_ _ _ w598 _ w671 _]
                seq-local: [_ _ w471 _ _ _ _] -> [_ _ _ w603 _ _ _]
                seq-local: [_ _ w466 _ _ _ _] -> [_ _ _ w600 _ _ _]
                seq-local: [w445 _ _ _ _ _ _] -> [_ _ w463 _ _ _ _]
                seq-local: [w444 _ _ _ _ _ _] -> [_ _ w462 _ _ _ _]
                seq-local: [_ _ w461 _ _ _ _] -> [_ _ _ _ w613 w675 _]
                seq-local: [_ _ _ w601 _ _ _] -> [_ _ _ _ w616 w663 _]
                seq-local: [_ _ _ w599 _ _ _] -> [_ _ _ _ _ w673 _]
                seq-local: [_ _ _ _ w612 _ _] -> [_ _ _ _ _ _ _]
                seq-local: [_ _ _ _ w610 _ _] -> [_ _ _ _ _ w664 _]
                tunnel: w441 -> [_ _ w468 w602 _ w674 _]
                tunnel: w440 -> [_ _ w469 w590 w619 w676 _]
                tunnel: w439 -> [_ _ w470 w589 w618 w677 _]
                tunnel: w438 -> [_ _ _ _ _ w661 _]
                tunnel: w437 -> [_ _ _ w609 _ _ _]
                tunnel: w436 -> [_ _ w467 _ _ _ _]
                tunnel: [_ _ _ w599 _ _ _] -> w433
                tunnel: [_ _ w461 _ _ _ _] -> w435
                tunnel: [_ _ _ w601 _ _ _] -> w434
                tunnel: w432 -> [_ _ _ _ _ w672 _]
                tunnel: w430 -> [w442 _ w460 w592 w617 w662 w894]
                tunnel: [_ _ _ _ _ w670 _] -> w431
                tunnel: [_ _ _ _ _ w668 _] -> w429
                tunnel: w428 -> [_ _ _ w604 w615 w667 _]
                tunnel: w427 -> [_ _ _ _ _ _ _]
                tunnel: w426 -> [_ _ _ _ _ w666 _]
                tunnel: w425 -> [_ _ _ _ w614 w665 _]
                tunnel: w424 -> [_ _ _ _ _ w660 _]
                frame #0 {
                  # "generate initial aberration (aberr to correct)"
                  n173 = case shown="\"Manual \"" "Initial Zern Coeffs" {
                    tunnel: ["Zern index initial" w456] -> w445
                    tunnel: ["Zern coeffs initial" w455] -> w444
                    frame "Manual " {
                    }
                    frame "Random" {
                      # "generate random zernike index and coefficient arrays"
                      n174 = local read "idxType"() -> (w453:enum16{"Wyant", "ANSI"})
                      n175 = call "zerncoeffs_RDgenerator.vi"("Defocus"="Defocus", "Tilts"="Tilts", "idxType"=w453, "Density"="Density", "Aplitude"="Amplitude", "Max zern num"="Max zern num") -> ("Zern coeff"=w455:sgl[], "Zern index"=w456:i32[])  [unwired: 4 in]
                      "Zern index (random)" <- w456
                      "Zern coeffs (random)" <- w455
                    }
                  }
                  n176 = Increment(x=w442) -> (x+1=→"Current Exp Num":i32)
                }
                frame #1 {
                  # "read in offset command"
                  n177 = call-poly <vilib>:"Read From Spreadsheet File.vi"("format (%.3f)"="%.8f", "file path (dialog if empty)"="Offset command file") -> ("first row"=w457:dbl[])  [unwired: 5 in, 4 out]
                }
                frame #2 {
                  w480 = 0.0
                  # "ini zern coeff"
                  # "offset+ini command"
                  # "Zern coeff"
                  # "Zern index"
                  # "calculate the command:\nfor phase diversity"
                  n178 = Array Size(array="Index 2") -> (size(s)=w478:i32)
                  n179 = call-poly <vilib>:"Ramp Pattern.vi"("start"=w480, "end"=w480, "samples"=w478) -> ("Ramp Pattern"=w477:dbl[])  [unwired: 7 in, 1 out]
                  n180 = Build Array(w477, "Index 2", "Index 3", "Index 4", "Index 5") -> (w464:T6)
                  n181 = Build Array(w477, "Coeffs 2", "Coeffs 3", "Coeffs 4", "Coeffs 5") -> (w481:T6)
                  n182 = Transpose Matrix(1:w481) -> (0:w474:T6)
                  n183 = Transpose Matrix(1:w464) -> (0:w472:T6)
                  n184 = Array Size(array=w464) -> (size(s)=w465:i32[])
                  n185 = Index Array(array=w465, index=1) -> (element=w471:i32)
                  "# of Phase" <- w471
                  n186 = stacked-sequence {
                    seq-local: [w494 _ _] -> [_ w510 w576]
                    seq-local: [w495 _ _] -> [_ w504 _]
                    seq-local: [_ w503 _] -> [_ _ w573]
                    seq-local: [w493 _ _] -> [_ w502 _]
                    tunnel: w471 -> [_ w513 _]
                    tunnel: w463 -> [w500 _ _]
                    tunnel: w462 -> [w499 w505 _]
                    tunnel: w475 -> [w497 _ _]
                    tunnel: w472 -> [_ w512 _]
                    tunnel: w474 -> [_ w511 _]
                    tunnel: [_ w509 _] -> w473
                    tunnel: w470 -> [_ w507 w574]
                    tunnel: w469 -> [_ w508 w575]
                    tunnel: w468 -> [_ w506 _]
                    tunnel: w467 -> [w496 _ _]
                    tunnel: [_ _ w572] -> w466
                    tunnel: [w494 _ _] -> w461
                    tunnel: w460 -> [_ w501 w570]
                    frame #0 {
                      n187 = local read "interaction matrix file"() -> (w489:path)
                      n188 = local read "Initial haso file"() -> (w490:path)
                      n189 = local read "idxType"() -> (w492:enum16{"Wyant", "ANSI"})
                      n190 = local read "Haso configuration file"() -> (w491:path)
                      n191 = call "zern2command_test.vi"("Haso configuration file"=w491, "idxType"=w492, "Initial haso file"=w490, "error in (no error)"=w496, "interaction matrix file"=w489, "Zern coef in"=w499, "Zern index in"=w500) -> ("error out"=w495:errorcluster, "Zern coef out"=w493:sgl[], "Offset positions"=w498:sgl[])  [unwired: 2 in]
                      n192 = Add(x=w498, y=w497) -> (x+y=w494:dbl[])
                    }
                    frame #1 {
                      n193 = for {
                        N: w513 -> [w516]
                        tunnel: w512 -> [w527] mode=indexing
                        tunnel: w511 -> [w526] mode=indexing
                        tunnel: w510 -> [w525]
                        tunnel: [w524] -> w509 mode=indexing
                        tunnel: w508 -> [w523]
                        tunnel: w507 -> [w522]
                        tunnel: w506 -> [w521]
                        tunnel: w505 -> [w520]
                        tunnel: w504 -> [w519]
                        tunnel: [w518] -> w503
                        tunnel: w502 -> [w515]
                        tunnel: w501 -> [w514]
                        i -> [w517]
                        n194 = stacked-sequence {
                          seq-local: [w537 _] -> [_ w548]
                          seq-local: [w533 _] -> [_ w556]
                          tunnel: w527 -> [w544 _]
                          tunnel: w526 -> [w543 _]
                          tunnel: w525 -> [w541 _]
                          tunnel: [w540 _] -> w524
                          tunnel: w523 -> [_ w558]
                          tunnel: w522 -> [_ w557]
                          tunnel: w521 -> [_ _]
                          tunnel: w517 -> [w539 _]
                          tunnel: w520 -> [w535 _]
                          tunnel: w519 -> [w534 _]
                          tunnel: [_ w555] -> w518
                          tunnel: w517 -> [_ _]
                          tunnel: w516 -> [_ _]
                          tunnel: w515 -> [w532 _]
                          tunnel: w514 -> [_ w552]
                          frame #0 {
                            n195 = Equal To 0?(x=w539) -> (x = 0?=w538:bool)
                            n196 = local read "idxType"() -> (w531:enum16{"Wyant", "ANSI"})
                            n197 = local read "Initial haso file"() -> (w529:path)
                            n198 = local read "interaction matrix file"() -> (w528:path)
                            n199 = local read "Haso configuration file"() -> (w530:path)
                            n200 = call "zern2command_test.vi"("Haso configuration file"=w530, "idxType"=w531, "Initial haso file"=w529, "error in (no error)"=w534, "interaction matrix file"=w528, "Zern coef in"=w543, "Zern index in"=w544) -> ("error out"=w533:errorcluster, "Zern coef out"=w536:sgl[], "Offset positions"=w542:sgl[])  [unwired: 2 in]
                            n201 = case shown="True" w538 {
                              tunnel: [w545 w546] -> w537
                              tunnel: w536 -> [w545 _]
                              tunnel: w535 -> [_ _]
                              tunnel: w532 -> [_ w546]
                              frame False {
                              }
                              frame True {
                              }
                            }
                            n202 = Add(x=w541, y=w542) -> (x+y=w540:dbl[])
                          }
                          frame #1 {
                            n203 = Number To Fractional String(number=w552, precision (6)=0) -> (F-format string=w551:string)  [unwired: 2 in]
                            n204 = Concatenate Strings(w558, w557, "_", w551, "_coeff.txt") -> (w566:string)
                            n205 = String To Path(string=w566) -> (path=w565:path)
                            n206 = Multiply(x=w548, y=1.0) -> (x*y=w547:dbl[])
                            n207 = Open/Create/Replace File(file path (use dialog)=w565, error in=w556, operation (0:open)=3) -> (refnum out=w562:refnum<file>, error out=w563:errorcluster)  [unwired: 3 in, 1 out]
                            n208 = Array To Spreadsheet String(array=w547, 3:"%f") -> (spreadsheet string=w554:string)  [unwired: 1 in]
                            n209 = Set File Position(refnum=w562, from (0:start)=1, error in=w563) -> (refnum out=w560:refnum<file>, error out=w559:errorcluster)  [unwired: 1 in]
                            n210 = Write to Text File(file (use dialog)=w560, text=w554, error in=w559) -> (error out=w555:errorcluster)  [unwired: 1 in, 2 out]
                          }
                        }
                      }
                    }
                    frame #2 {
                      n211 = Number To Fractional String(number=w570, precision (6)=0) -> (F-format string=w569:string)  [unwired: 2 in]
                      n212 = Concatenate Strings(w575, w574, "_", w569, "_IniAbr+offset.txt") -> (w585:string)
                      n213 = String To Path(string=w585) -> (path=w583:path)
                      n214 = Open/Create/Replace File(file path (use dialog)=w583, error in=w573, operation (0:open)=3) -> (refnum out=w580:refnum<file>, error out=w581:errorcluster)  [unwired: 3 in, 1 out]
                      n215 = Array To Spreadsheet String(array=w576, 3:"%f") -> (spreadsheet string=w587:string)  [unwired: 1 in]
                      n216 = Set File Position(refnum=w580, from (0:start)=1, error in=w581) -> (refnum out=w578:refnum<file>, error out=w577:errorcluster)  [unwired: 1 in]
                      n217 = Write to Text File(file (use dialog)=w578, text=w587, error in=w577) -> (error out=w572:errorcluster)  [unwired: 1 in, 2 out]
                    }
                  }
                }
                frame #3 {
                  # "save phase diversity pictures:\npictures per phase*number of phases (Eg: 2*5=10 pictures in this file)"
                  # "readout and delay"
                  # "take phase diversity pictures"
                  n218 = local read "EMCCD trigger port"() -> (w605:tag)
                  n219 = Number To Fractional String(number=w592, precision (6)=0) -> (F-format string=w596:string)  [unwired: 2 in]
                  n220 = Multiply(x=w609, y=1000.0) -> (x*y=w608:dbl)
                  n221 = Concatenate Strings(w590, w589, "_", w596) -> (w591:string)
                  n222 = Add(x=w608, y=50.0) -> (x+y=w601:dbl)
                  n223 = call "applyDM_and_acqTIFF_mCMD.vi"("EMCCD trigger port"=w605, "WavefrontCorrector in"=w604, "Absolute Positions"=w598, "exp and readout time (ms)"=w601, "CMD Num"=w603, "Img Num"=w602, "error in (no error)"=w600, "strPath"=w591, "Clean Spooling"=TRUE, "strPalette"="C:\\Program Files\\Andor SOLIS\\GREY.PAL") -> ("error out"=w599:errorcluster)  [unwired: 4 in, 1 out]
                }
                frame #4 {
                  # "take a picture of groundtruth and offset+ini abbr, and cal imq for each"
                  n224 = stacked-sequence {
                    tunnel: w619 -> [w634 w653]
                    tunnel: w618 -> [w633 w652]
                    tunnel: w617 -> [w632 w651]
                    tunnel: w616 -> [w628 w648]
                    tunnel: w613 -> [_ w640]
                    tunnel: w615 -> [w631 w650]
                    tunnel: w614 -> [w621 w642]
                    tunnel: [w620 _] -> w612
                    tunnel: w611 -> [w630 _]
                    tunnel: [_ w638] -> w610
                    frame #0 {
                      # "calculate imq of groundtruth"
                      # "take a picture of groundtruth"
                      n225 = Number To Fractional String(number=w632, precision (6)=0) -> (F-format string=w635:string)  [unwired: 2 in]
                      n226 = Concatenate Strings(w634, w633, "_grdtrth_", w635) -> (w624:string)
                      n227 = local read "EMCCD trigger port"() -> (w629:tag)
                      n228 = call "applyDM_and_acqTIFF.vi"("EMCCD trigger port"=w629, "WavefrontCorrector in"=w631, "Absolute Positions"=w630, "exp and readout time (ms)"=w628, "Img Num"=1, "strPath"=w624) -> ("error out"=w625:errorcluster)  [unwired: 8 in, 1 out]
                      n229 = Concatenate Strings(w624, ".tif") -> (w623:string)
                      n230 = call "calculate_IQM_MATLAB.vi"("error in (no error)"=w625, "Background Value"=w621, "File Path and Name w/.tif"=w623, "Metrics Type"="Metrics Type") -> ("image quality"=w620:dbl)  [unwired: 6 in, 1 out]
                      "Groundtruth IQM" <- w620
                    }
                    frame #1 {
                      # "take a picture of offset+ini abbr"
                      # "calculate imq of groundtruth"
                      n231 = Number To Fractional String(number=w651, precision (6)=0) -> (F-format string=w654:string)  [unwired: 2 in]
                      n232 = Concatenate Strings(w653, w652, "_abbr_", w654) -> (w644:string)
                      n233 = local read "EMCCD trigger port"() -> (w649:tag)
                      n234 = call "applyDM_and_acqTIFF.vi"("EMCCD trigger port"=w649, "WavefrontCorrector in"=w650, "Absolute Positions"=w640, "exp and readout time (ms)"=w648, "Img Num"=1, "strPath"=w644) -> ("error out"=w645:errorcluster)  [unwired: 8 in, 1 out]
                      n235 = Concatenate Strings(w644, ".tif") -> (w643:string)
                      n236 = local read "Metrics Type"() -> (w641:T4)
                      n237 = call "calculate_IQM_MATLAB.vi"("error in (no error)"=w645, "Background Value"=w642, "File Path and Name w/.tif"=w643, "Metrics Type"=w641) -> ("image quality"=w638:dbl)  [unwired: 6 in, 1 out]
                      "Aberrated IQM" <- w638
                    }
                  }
                }
                frame #5 {
                  # "run matlab correction?"
                  n238 = local read "interaction matrix file"() -> (w659:path)
                  n239 = local read "Initial haso file"() -> (w658:path)
                  n240 = local read "Haso configuration file"() -> (w657:path)
                  n241 = case shown="True" w672 {
                    tunnel: w676 -> [_ w704]
                    tunnel: w677 -> [_ w703]
                    tunnel: w675 -> [_ w702]
                    tunnel: w663 -> [_ w701]
                    tunnel: w674 -> [_ w700]
                    tunnel: w673 -> [_ w699]
                    tunnel: w662 -> [_ w698]
                    tunnel: w671 -> [_ _]
                    tunnel: [0 w697] -> w670
                    tunnel: w669 -> [_ w696]
                    tunnel: [errorcluster {"status"=FALSE, "code"=0, "source"=""} ("Error out 2") w695] -> w668
                    tunnel: w667 -> [_ w694]
                    tunnel: w666 -> [_ w693]
                    tunnel: w665 -> [_ w692]
                    tunnel: w664 -> [_ w689]
                    tunnel: w663 -> [_ w691]
                    tunnel: w662 -> [_ w690]
                    tunnel: w661 -> [_ w688]
                    tunnel: w660 -> [_ w687]
                    tunnel: w659 -> [_ w685]
                    tunnel: w658 -> [_ w684]
                    tunnel: w657 -> [_ w683]
                    tunnel: "Initial Phase Num" -> [_ w682]
                    frame False {
                      n242 = local write "All IQM"(dbl[] []) -> ()
                    }
                    frame True {
                      # "matlab reconstructed Zern"
                      n243 = stacked-sequence {
                        seq-local: [w721 _] -> [_ w847]
                        seq-local: [w723 _] -> [_ w846]
                        tunnel: w704 -> [w722 w866]
                        tunnel: w703 -> [w720 w865]
                        tunnel: w702 -> [w715 w852]
                        tunnel: w701 -> [_ _]
                        tunnel: w699 -> [_ _]
                        tunnel: w700 -> [_ _]
                        tunnel: w698 -> [w719 w864]
                        tunnel: [w718 _] -> w697
                        tunnel: w696 -> [_ w857]
                        tunnel: [_ w844] -> w695
                        tunnel: w694 -> [w710 w850]
                        tunnel: w693 -> [_ _]
                        tunnel: w692 -> [w717 _]
                        tunnel: w691 -> [w714 w858]
                        tunnel: w690 -> [w713 _]
                        tunnel: w682 -> [w716 _]
                        tunnel: w689 -> [w712 _]
                        tunnel: w688 -> [w711 _]
                        tunnel: w687 -> [_ _]
                        tunnel: [w709 _] -> w686
                        tunnel: w685 -> [w708 w848]
                        tunnel: w684 -> [w707 w843]
                        tunnel: w683 -> [w706 w842]
                        tunnel: [w705 _] -> w681
                        frame #0 {
                          n244 = while {
                            tunnel: [w746] -> w723
                            tunnel: w722 -> [w745]
                            tunnel: [w744] -> w721
                            tunnel: w720 -> [w743]
                            tunnel: w719 -> [w742]
                            tunnel: [w741] -> w718
                            tunnel: w717 -> [w740]
                            shift-right: [w732] -> _
                            shift-left: w716 -> [w739]
                            tunnel: w715 -> [w738]
                            tunnel: w714 -> [w737]
                            tunnel: w713 -> [w736]
                            tunnel: w712 -> [w735]
                            tunnel: w711 -> [w730]
                            tunnel: w710 -> [w729]
                            tunnel: [w728] -> w709 mode=indexing
                            tunnel: w708 -> [w727]
                            tunnel: w707 -> [w726]
                            tunnel: w706 -> [w725]
                            tunnel: [w724] -> w705 mode=indexing
                            stop <- w733 stop-if-true
                            n245 = stacked-sequence {
                              seq-local: [w759 _ _] -> [_ w803 _]
                              seq-local: [w758 _ _] -> [_ w811 _]
                              tunnel: [w758 _ _] -> w746
                              tunnel: w745 -> [w777 w813 _]
                              tunnel: [w759 _ _] -> w744
                              tunnel: w743 -> [w756 w812 _]
                              tunnel: w742 -> [w771 _ _]
                              tunnel: [w750 _ _] -> w741
                              tunnel: w740 -> [w760 w790 _]
                              tunnel: w739 -> [w747 w808 w829]
                              tunnel: w738 -> [_ w810 _]
                              tunnel: w737 -> [_ w798 _]
                              tunnel: w736 -> [_ w809 _]
                              tunnel: w735 -> [_ w788 _]
                              tunnel: [_ w791 _] -> w734
                              tunnel: [_ _ w828] -> w732
                              tunnel: [_ _ w827] -> w731
                              tunnel: w730 -> [_ _ _]
                              tunnel: w729 -> [_ w801 _]
                              tunnel: [_ w786 _] -> w728
                              tunnel: w727 -> [_ w806 _]
                              tunnel: w726 -> [_ w805 _]
                              tunnel: w725 -> [_ w804 _]
                              tunnel: [w747 _ _] -> w724
                              frame #0 {
                                w753 = "_"
                                n246 = local read "idxType"() -> (w749:enum16{"Wyant", "ANSI"})
                                n247 = Number To Fractional String(number=w771, precision (6)=0) -> (F-format string=w752:string)  [unwired: 2 in]
                                n248 = Concatenate Strings(w756, "_", w752) -> (w761:string)
                                n249 = String To Path(string=w777) -> (path=w778:path)
                                n250 = Number To Fractional String(number=w747, precision (6)=0) -> (F-format string=w755:string)  [unwired: 2 in]
                                n251 = Concatenate Strings(w777, w756, w753, w755, "ImgCorr", w753, w752) -> (w776:string)
                                n252 = case shown="\"ANSI\"" w749 {
                                tunnel: [2 3] -> w748
                                frame "Wyant", Default {
                                }
                                frame "ANSI" {
                                }
                                }
                                n253 = String To Path(string=w776) -> (path=w775:path)
                                n254 = call "recon_zern_fileIO_MATLAB_v2.vi"("Number of Phase"=w747, "Number for average"="Num for average", "Crop Size of image"="Crop Size of image", "Background Value"=w760, "Zernike Order"="Zernike Index Limit", "Use GPU"="Use GPU", "Iteration Number"="Max Iteration Num", "idxType"=w749, "File Name"=w761, "Gamma Value"="Gamma Value", "Path In"=w778, "Show Input"="Show Input", "Path Out"=w775, "Show Recon"="Show Recon") -> ("Zern coef out"=w773:sgl[], "Time cost (s)"=→"Recon Time (s)":dbl, "RMSE Value"=w750:dbl, "error out"=w758:errorcluster)  [unwired: 10 in]
                                "RMSE Value" <- w750
                                n255 = case shown="True" "Apply Defocus" {
                                tunnel: w773 -> [w781 w785]
                                tunnel: [w781 w783] -> w759
                                tunnel: w748 -> [_ w782]
                                frame False {
                                }
                                frame True {
                                n256 = Replace Array Subset(array=w785, new element=0.0, index=w782) -> (w783:sgl[])
                                }
                                }
                                "Recon Img Num" <- w747
                              }
                              frame #1 {
                                w821 = 1
                                # "get correction command\ntake a picture"
                                n257 = Number To Fractional String(number=w808, precision (6)=0) -> (F-format string=w814:string)  [unwired: 2 in]
                                n258 = Array Size(array=w803) -> (size(s)=w802:i32)
                                n259 = Number To Fractional String(number=w809, precision (6)=0) -> (F-format string=w817:string)  [unwired: 2 in]
                                n260 = call-poly <vilib>:"Ramp Pattern.vi"("start"=w821, "end"=w802, "delta"=w821) -> ("Ramp Pattern"=w820:dbl[])  [unwired: 6 in, 2 out]
                                n261 = Concatenate Strings(w813, w812, "_", w814, "ImgCorr_", w817) -> (w792:string)
                                n262 = local read "idxType"() -> (w807:enum16{"Wyant", "ANSI"})
                                n263 = call "zern2command_test.vi"("Haso configuration file"=w804, "idxType"=w807, "Initial haso file"=w805, "error in (no error)"=w811, "interaction matrix file"=w806, "Zern coef in"=w803, "Zern index in"=w820) -> ("error out"=w793:errorcluster, "Offset positions"=w819:sgl[])  [unwired: 2 in, 1 out]
                                n264 = Add(x=w810, y=w819) -> (x+y=w799:dbl[])
                                n265 = call "applyDM_and_acqTIFF.vi"("WavefrontCorrector in"=w801, "Absolute Positions"=w799, "exp and readout time (ms)"=w798, "Img Num"=1, "error in (no error)"=w793, "strPath"=w792) -> ("error out"=w789:errorcluster)  [unwired: 8 in, 1 out]
                                n266 = Concatenate Strings(w792, ".tif") -> (w797:string)
                                n267 = local read "Metrics Type"() -> (w796:T4)
                                n268 = call "calculate_IQM_MATLAB.vi"("error in (no error)"=w789, "Background Value"=w790, "File Path and Name w/.tif"=w797, "Metrics Type"=w796) -> ("image quality"=w786:dbl)  [unwired: 6 in, 1 out]
                                "Corrected IQM" <- w786
                                n269 = case shown="True" "Auto Stop" {
                                tunnel: [FALSE w825] -> w791
                                tunnel: w786 -> [_ w824]
                                tunnel: w788 -> [_ w823]
                                frame False {
                                }
                                frame True {
                                n270 = Greater?(x=w824, y=w823) -> (0:w825:bool)
                                }
                                }
                              }
                              frame #2 {
                                n271 = case shown="\"Progressive Feedback\"" "Feedback Type" {
                                tunnel: w829 -> [w832 w834 w836]
                                tunnel: [w832 w833 w837] -> w828
                                tunnel: [TRUE w835 w839] -> w827
                                tunnel: "Final Phase Num" -> [_ w833 w838]
                                frame "Single Correction", Default {
                                }
                                frame "One Step Feedback" {
                                n272 = Greater Or Equal?(x=w834, y=w833) -> (x >= y?=w835:bool)
                                }
                                frame "Progressive Feedback" {
                                n273 = Increment(x=w836) -> (x+1=w837:u32)
                                n274 = Greater Or Equal?(x=w836, y=w838) -> (x >= y?=w839:bool)
                                }
                                }
                              }
                            }
                            n275 = Or(x=w734, y=w731) -> (x .or. y?=w733:bool)
                          }
                        }
                        frame #1 {
                          w856 = 1
                          # "set andor kinetics and spooling, \nstart acquire and wait for the external trigger"
                          n276 = Array Size(array=w847) -> (size(s)=w853:i32)
                          n277 = call-poly <vilib>:"Ramp Pattern.vi"("start"=w856, "end"=w853, "delta"=w856) -> ("Ramp Pattern"=w855:dbl[])  [unwired: 6 in, 2 out]
                          n278 = local read "idxType"() -> (w849:enum16{"Wyant", "ANSI"})
                          n279 = call "zern2command_test.vi"("Haso configuration file"=w842, "idxType"=w849, "Initial haso file"=w843, "error in (no error)"=w846, "interaction matrix file"=w848, "Zern coef in"=w847, "Zern index in"=w855) -> ("error out"=w845:errorcluster, "Offset positions"=w854:sgl[])  [unwired: 2 in, 1 out]
                          n280 = Add(x=w852, y=w854) -> (x+y=w851:dbl[])
                          n281 = Build Array(w857, w852, w851) -> (w841:T6)
                          n282 = Number To Fractional String(number=w864, precision (6)=0) -> (F-format string=w867:string)  [unwired: 2 in]
                          n283 = Transpose Matrix(1:w841) -> (0:w840:T6)
                          n284 = local read "EMCCD trigger port"() -> (w859:tag)
                          n285 = Concatenate Strings(w866, w865, "_grdtrth_abrr_Corr_", w867) -> (w863:string)
                          n286 = call "applyDM_and_acqTIFF_mCMD.vi"("EMCCD trigger port"=w859, "WavefrontCorrector in"=w850, "Absolute Positions"=w840, "exp and readout time (ms)"=w858, "CMD Num"=3, "Img Num"=1, "error in (no error)"=w845, "strPath"=w863) -> ("error out"=w844:errorcluster)  [unwired: 6 in, 1 out]
                        }
                      }
                      "All IQM" <- w686
                      "Img Num Used" <- w681
                    }
                  }
                }
                frame #6 {
                  # "save image quality values"
                  n287 = local read "File Base Name"() -> (w876:string)
                  n288 = local read "Output path"() -> (w877:path)
                  n289 = Number To Fractional String(number=w894, precision (6)=0) -> (F-format string=w883:string)  [unwired: 2 in]
                  n290 = Concatenate Strings(w883, ".txt") -> (w874:string)
                  n291 = local read "Img Num Used"() -> (w893:dbl[])
                  n292 = local read "All IQM"() -> (w892:dbl[])
                  n293 = local read "Groundtruth IQM"() -> (w891:dbl)
                  n294 = local read "Aberrated IQM"() -> (w890:dbl)
                  n295 = Concatenate Strings(w876, "_IQM_InitialAber_", w874) -> (w882:string)
                  n296 = Build Array(w893, w892) -> (w878:T6)
                  n297 = Concatenate Strings(w876, "_IQM_Corrected_", w874) -> (w873:string)
                  n298 = Build Array(w891, w890) -> (w886:dbl[])
                  n299 = Build Path(base path=w877, name or relative path=w882) -> (appended path=w887:path)
                  n300 = Array To Spreadsheet String(array=w886, 3:"%f") -> (spreadsheet string=w888:string)  [unwired: 1 in]
                  n301 = Build Path(base path=w877, name or relative path=w873) -> (appended path=w879:path)
                  n302 = Array To Spreadsheet String(array=w878, 3:"%f") -> (spreadsheet string=w880:string)  [unwired: 1 in]
                  n303 = Write to Text File(file (use dialog)=w887, text=w888) -> (refnum out=w870:refnum<file>, error out=w869:errorcluster)  [unwired: 2 in, 1 out]
                  n304 = Write to Text File(file (use dialog)=w879, text=w880) -> (refnum out=w872:refnum<file>, error out=w871:errorcluster)  [unwired: 2 in, 1 out]
                  n305 = Close File(refnum=w870, error in=w869) -> ()  [unwired: 2 out]
                  n306 = Close File(refnum=w872, error in=w871) -> ()  [unwired: 2 out]
                }
              }
            }
          }
          frame #2 {
            # "shut down shutter of 488nm laser"
            n307 = invoke class="MG17Motor" method="SC_Disable"(reference=w899, "lChanID"=w898) -> (reference out=w897:refnum<k7>, "lChanID"=w896:i32)  [unwired: 2 in, 2 out]
          }
          frame #3 {
            # "save the RMS of (calculated zer-real zer)"
            n308 = Concatenate Strings(w902, w901, "_RMSE.txt") -> (w907:string)
            n309 = String To Path(string=w907) -> (path=w906:path)
            n310 = Number To Fractional String(number=w903) -> (F-format string=w904:string[])  [unwired: 3 in]
            n311 = Write to Text File(file (use dialog)=w906, text=w904) -> (error out=w900:errorcluster)  [unwired: 2 in, 2 out]
          }
        }
        n312 = Merge Errors(w381, w380, w375) -> (w374:errorcluster)
        "Error out" <- w374
        n313 = Unbundle(w374) -> ("status"=w370:bool)  [unwired: 2 out]
        n314 = case shown="False" w370 {
          tunnel: [w395 w396] -> w373
          tunnel: w370 -> [w394 w396]
          frame False {
            n315 = Not(x=w394) -> (.not. x?=w395:bool)
          }
          frame True {
          }
        }
        n316 = Or(x=w373, y="?") -> (x .or. y?=w371:bool)
      }
    }
    frame #4 {
      n317 = case shown="True" "Turn off EMCCD when finished?" {
        frame False {
        }
        frame True {
          n318 = flat-sequence {
            frame #0 {
              n319 = call <userlib>:"CoolerOFF.vi"() -> ()  [unwired: 2 in, 2 out]
            }
            frame #1 {
              # "shut down EMCCD"
              n320 = call <userlib>:"ShutDown.vi"() -> ()  [unwired: 2 in, 2 out]
            }
          }
        }
      }
    }
    frame #5 {
      # "if not \"stop control\", the shutter can be control when the program is not running"
      # "shut down casao"
      n321 = call <userlib>:"LVClass_WavefrontCorrector dtor.vi"("WavefrontCorrector in"=w913, "error in (no error)"=w911) -> ("error out"=w910:errorcluster)  [unwired: 12 in, 1 out]
      n322 = call <userlib>:"LVClass_WavefrontCorrectorSet dtor.vi"("WavefrontCorrectorSet in"=w912, "error in (no error)"=w910) -> ()  [unwired: 12 in, 2 out]
      n323 = case shown="True" FALSE {
        tunnel: w914 -> [_ w915]
        frame False {
        }
        frame True {
          n324 = invoke class="MG17Motor" method="StopCtrl"(reference=w915) -> ()  [unwired: 2 in, 3 out]
        }
      }
    }
  }
  n325 = local read "Metrics Type"() -> (w1:T4)
  n326 = case shown="\"sharpness - image domain\"" w1 {
    tunnel: [" \" \", Default." " \"max intensity\"." " \"mean intensity\"." " \"RMS contrast\"." " \"sharpness - image domain\"." " \"sharpness - spectral domain 1: 0~r0\"." " \"sharpness - spectral domain 2: 0.1*r0~0.5*r0\"." " \"norm DCT  - spectral domain 3: 0~r0\"."] -> _
    frame " ", Default {
    }
    frame "max intensity" {
    }
    frame "mean intensity" {
    }
    frame "RMS contrast" {
    }
    frame "sharpness - image domain" {
    }
    frame "sharpness - spectral domain 1: 0~r0" {
    }
    frame "sharpness - spectral domain 2: 0.1*r0~0.5*r0" {
    }
    frame "norm DCT  - spectral domain 3: 0~r0" {
    }
  }
